vi "MSTAutoDailyReport.vi"() -> ()   [LabVIEW 2012]
uses:
  <vilib>/Utility/NIReport.llb/NI_report.lvclass
  <vilib>/addons/database/Connection.llb/DB Tools Open Connec (Path).vi
  <vilib>/addons/database/Connection.llb/Conn Execute.vi
  <vilib>/addons/database/Recordset.llb/Rec Fetch Recordset Data (R).vi
  <vilib>/addons/database/Recordset.llb/Rec Destroy - Connection.vi
  <vilib>/Utility/NIReport.llb/Append Text Table to Report (wrap).vi
  <vilib>/addons/database/_DB Variant To Data/Database Variant To Data.xnode
  <vilib>/addons/database/NI_Database_API.lvlib
  <vilib>/Utility/NIReport.llb/Excel/NI_Excel.lvclass
  <vilib>/addons/_office/NI_ReportGenerationToolkit.lvlib
panel:
  out "error out 3":errorcluster
  out "appended array 3":string[](array[string])
  out "recordset data 3":variant[][](array[variant])
  out "error out 5":errorcluster
  out "appended array 4":string[](array[string])
  out "recordset data 4":variant[][](array[variant])
  out "error out 6":errorcluster
  out "appended array 5":string[](array[string])
  out "recordset data 5":variant[][](array[variant])
  out "error out 4":errorcluster
  in  "Table Control 4":string[][](table)
  in  "Table Control 3":string[][](table)
  in  "Table Control 2":string[][](table)
  out "appended array":string[](array[string])
  out "recordset data":variant[][](array[variant])
  in  "Report Template":path=path "O:/Monitor/Report/MSTDailyReport.xls"
  in  "Table Control":string[][](table)
  out "error out":errorcluster
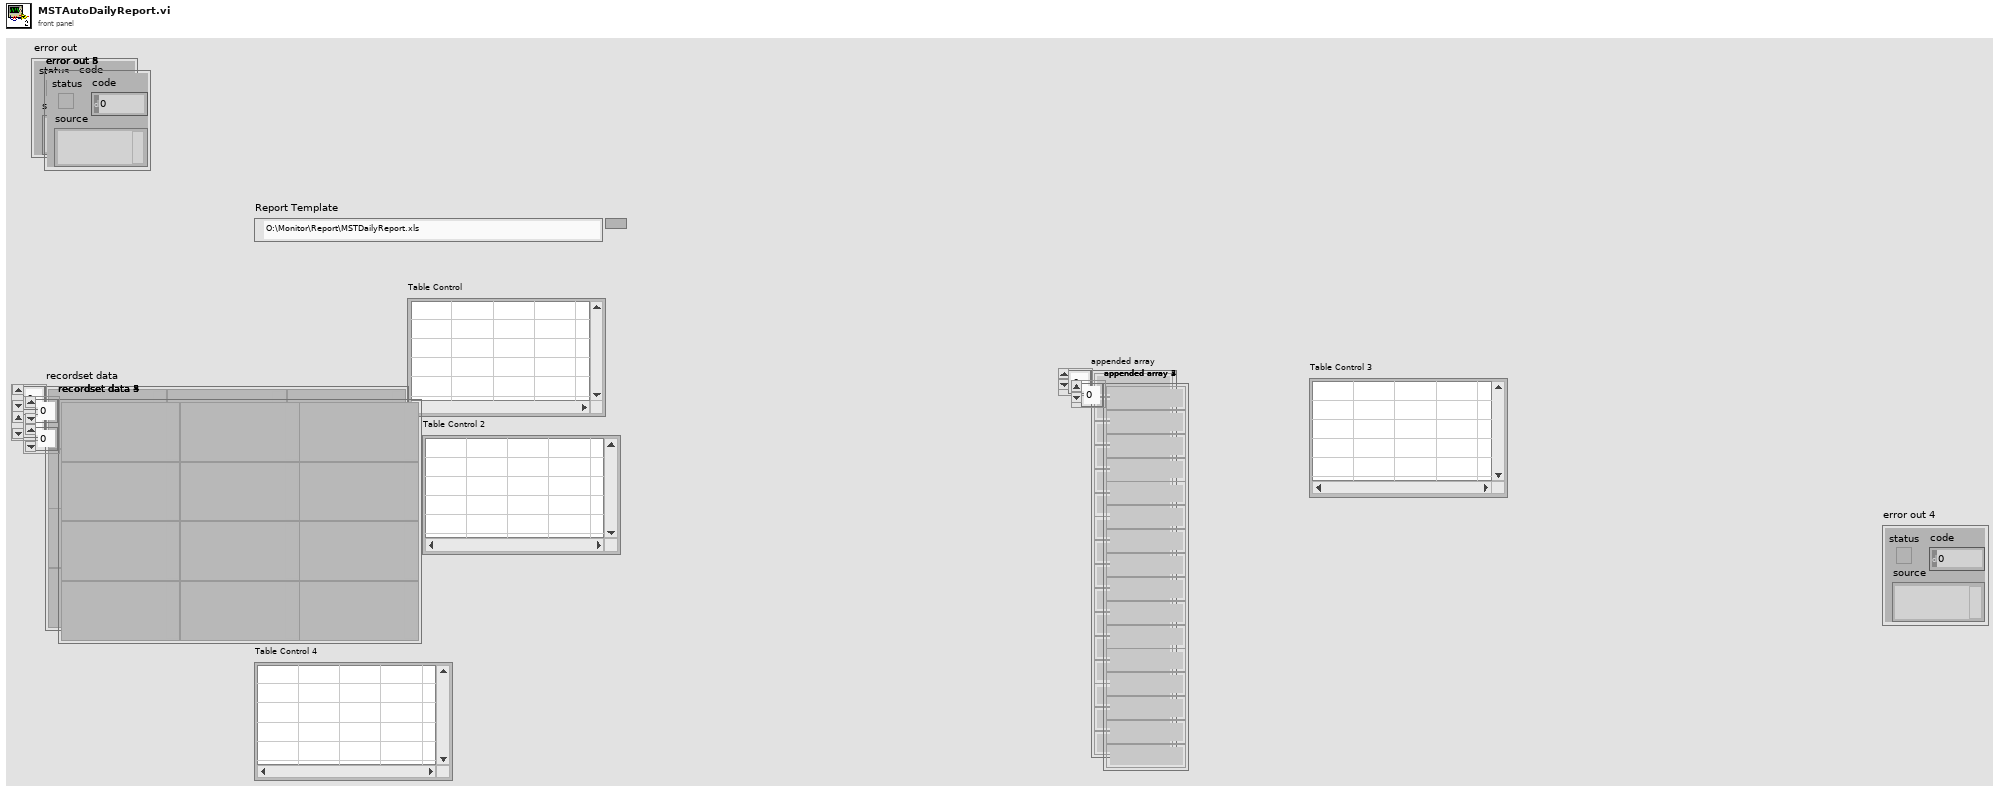
[diagram p1: front panel]
types:
  T1 = typedef "NI_Database_API.lvlib/Conn ObjectReference.ctl" = refnum<k1>
  T2 = typedef "NI_Database_API.lvlib/Rec ObjectReference.ctl" = refnum<k1>
  T3 = enum16{"Standard Report", "HTML", "Word", "Excel"}
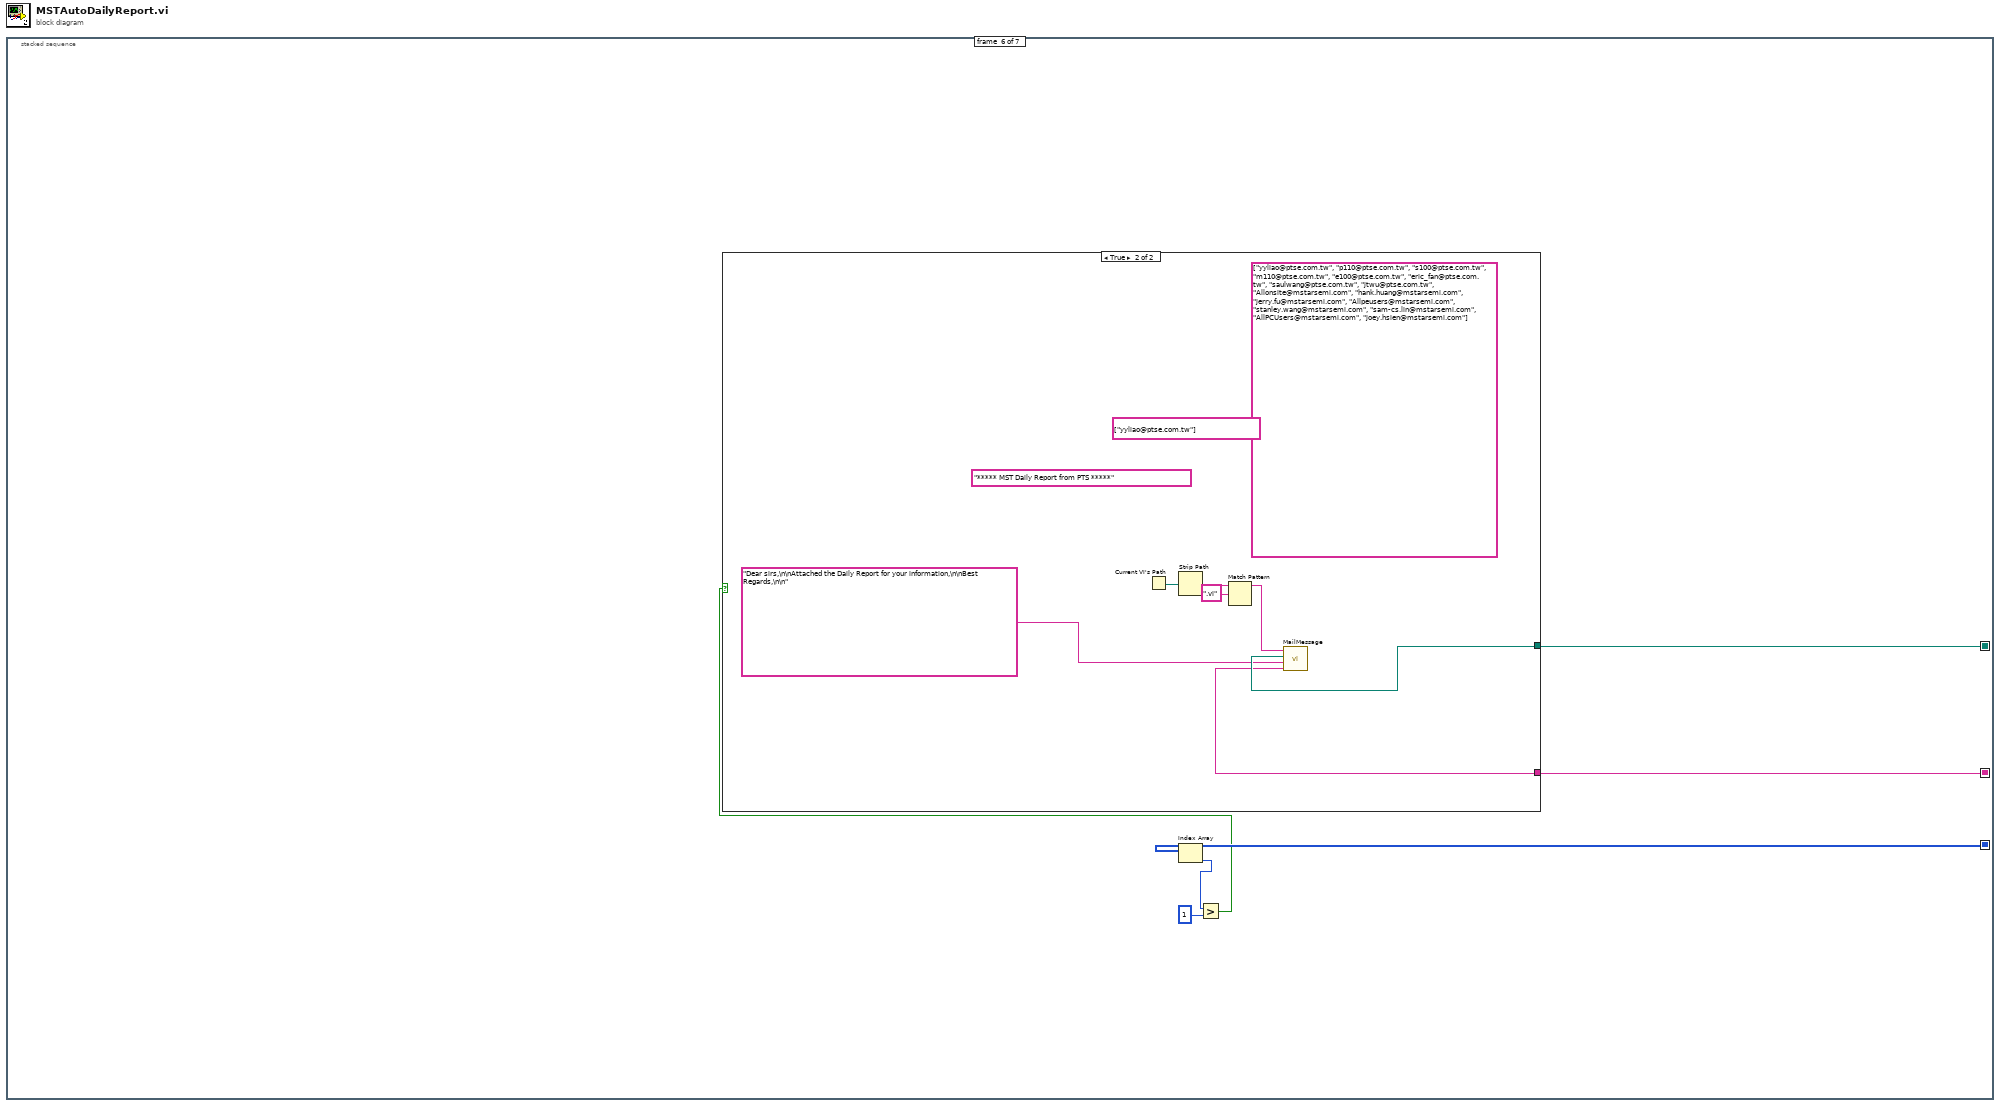
[diagram p0: block diagram]
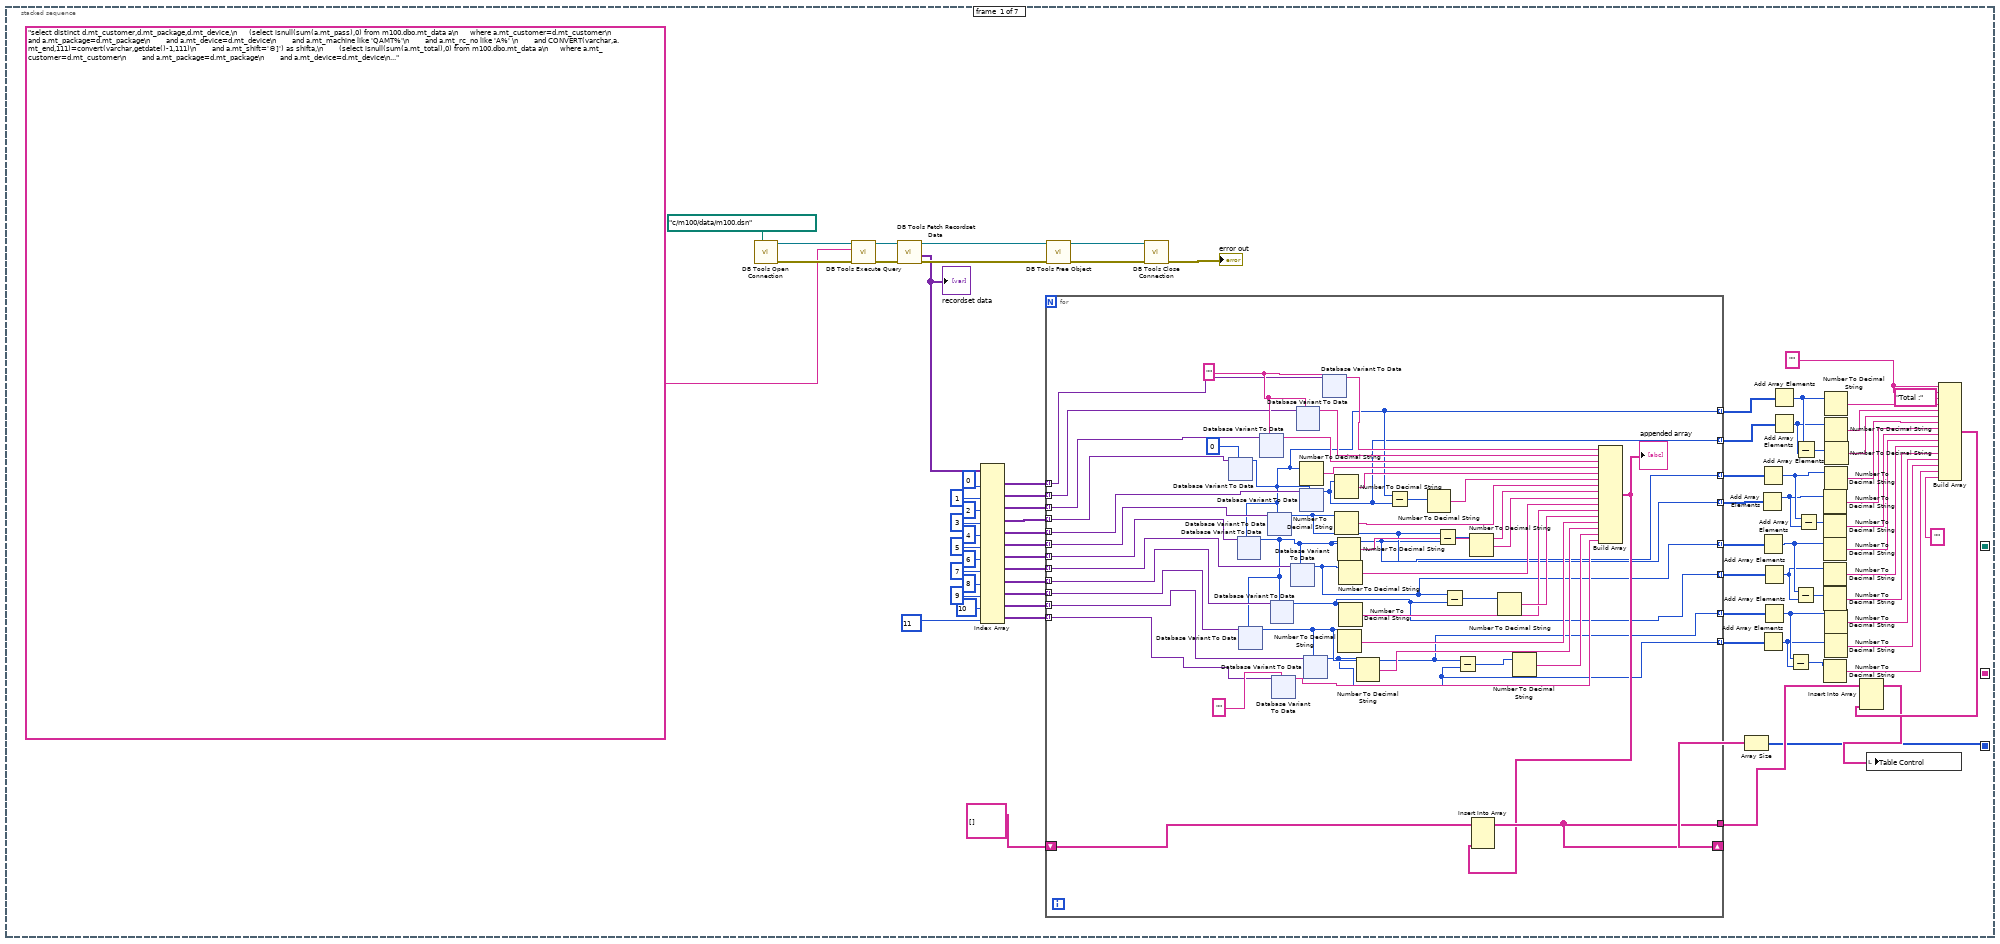
[diagram p2: hidden frame]
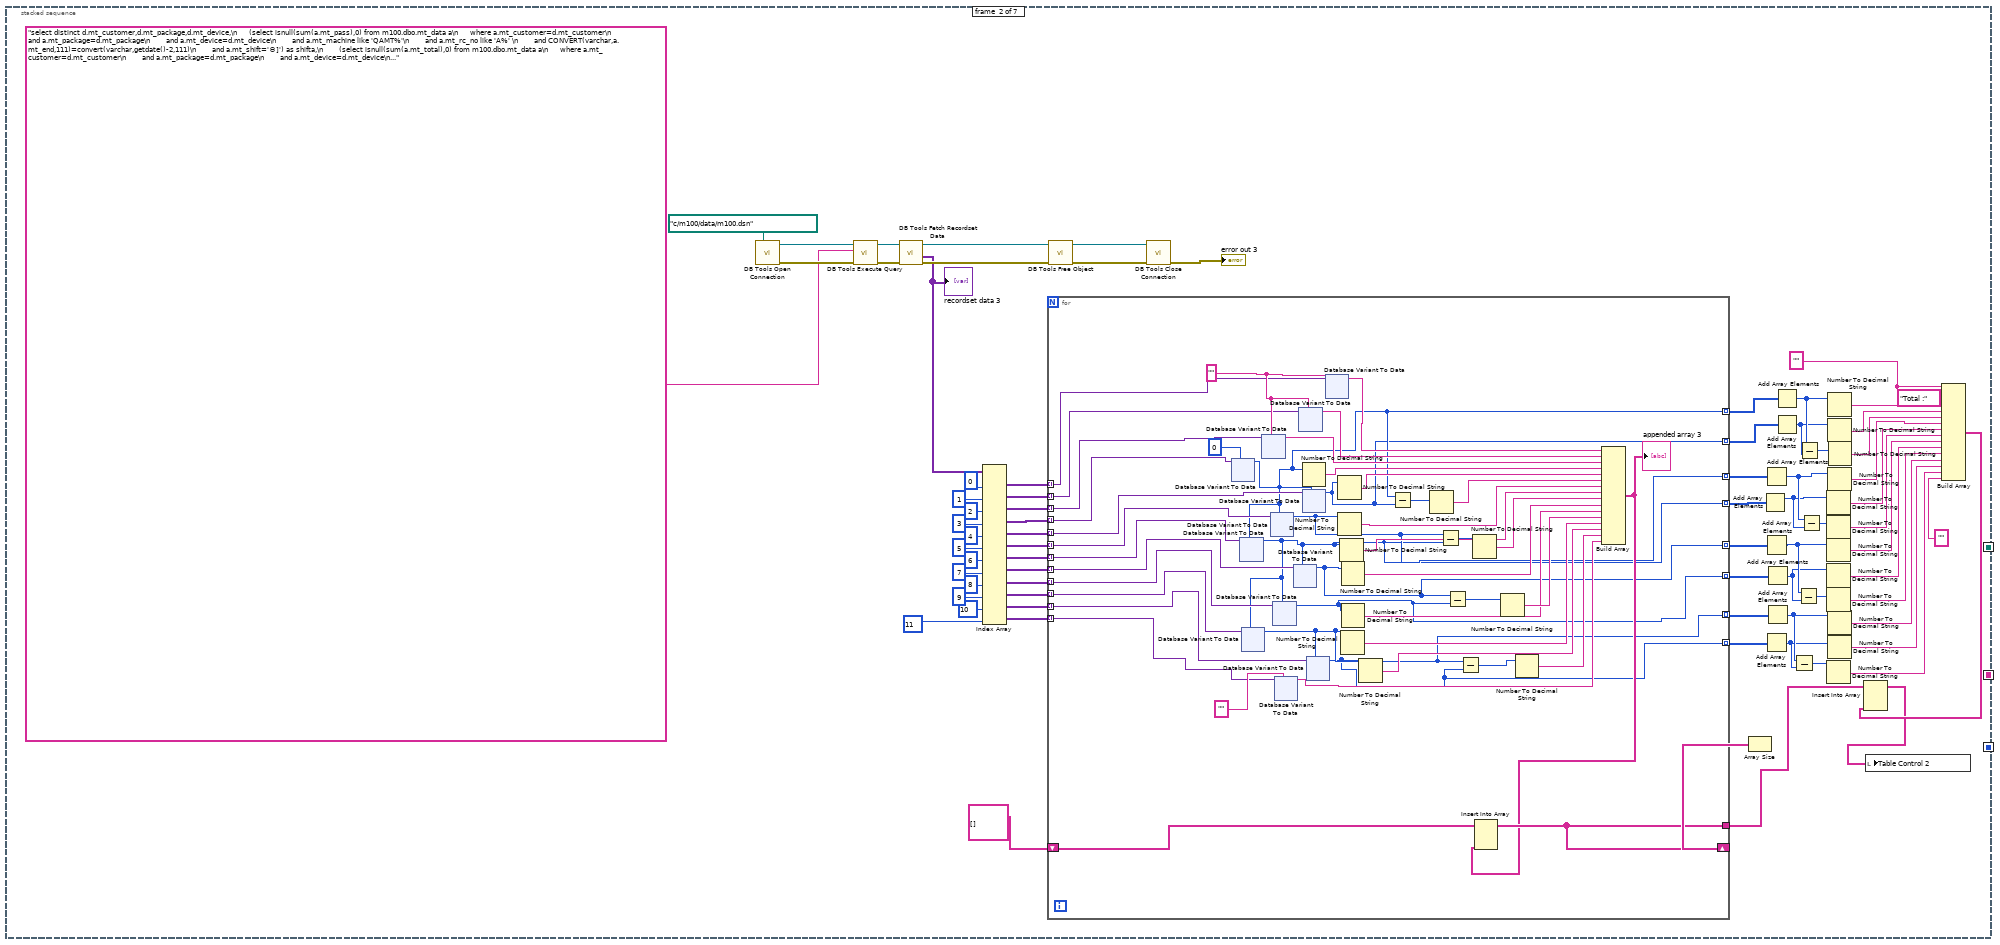
[diagram p3: hidden frame]
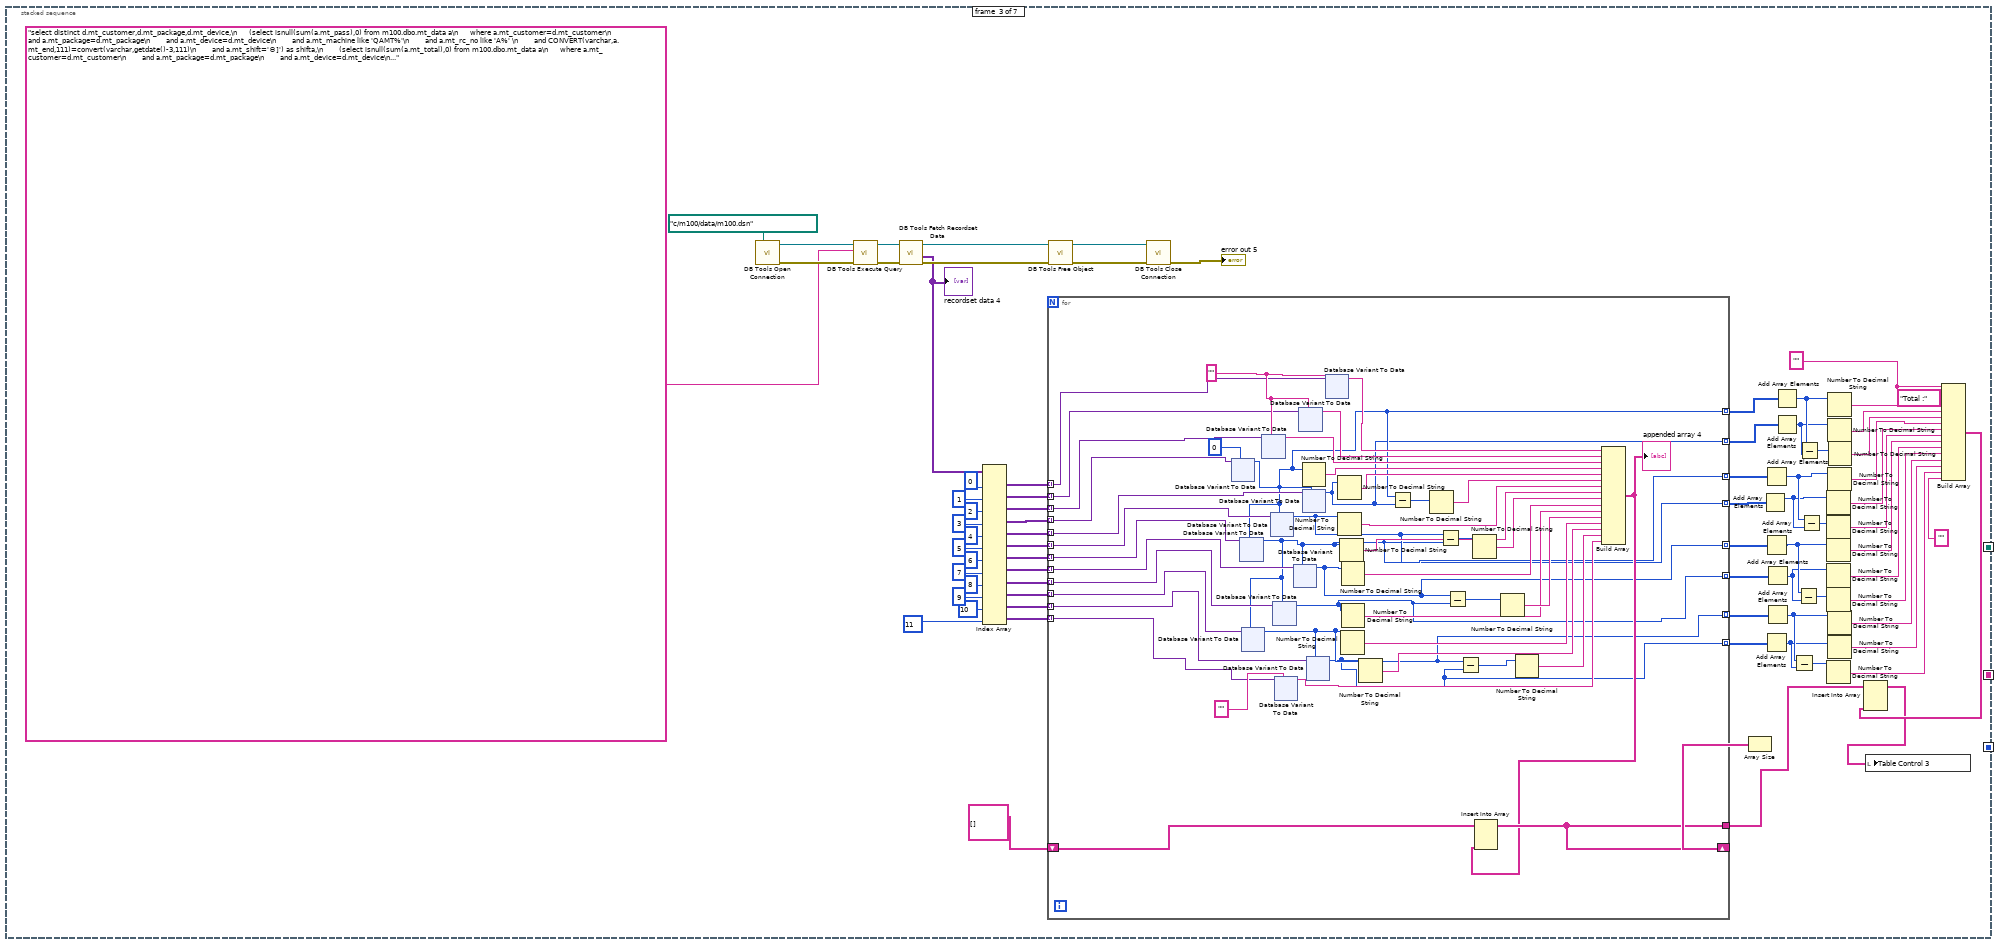
[diagram p4: hidden frame]
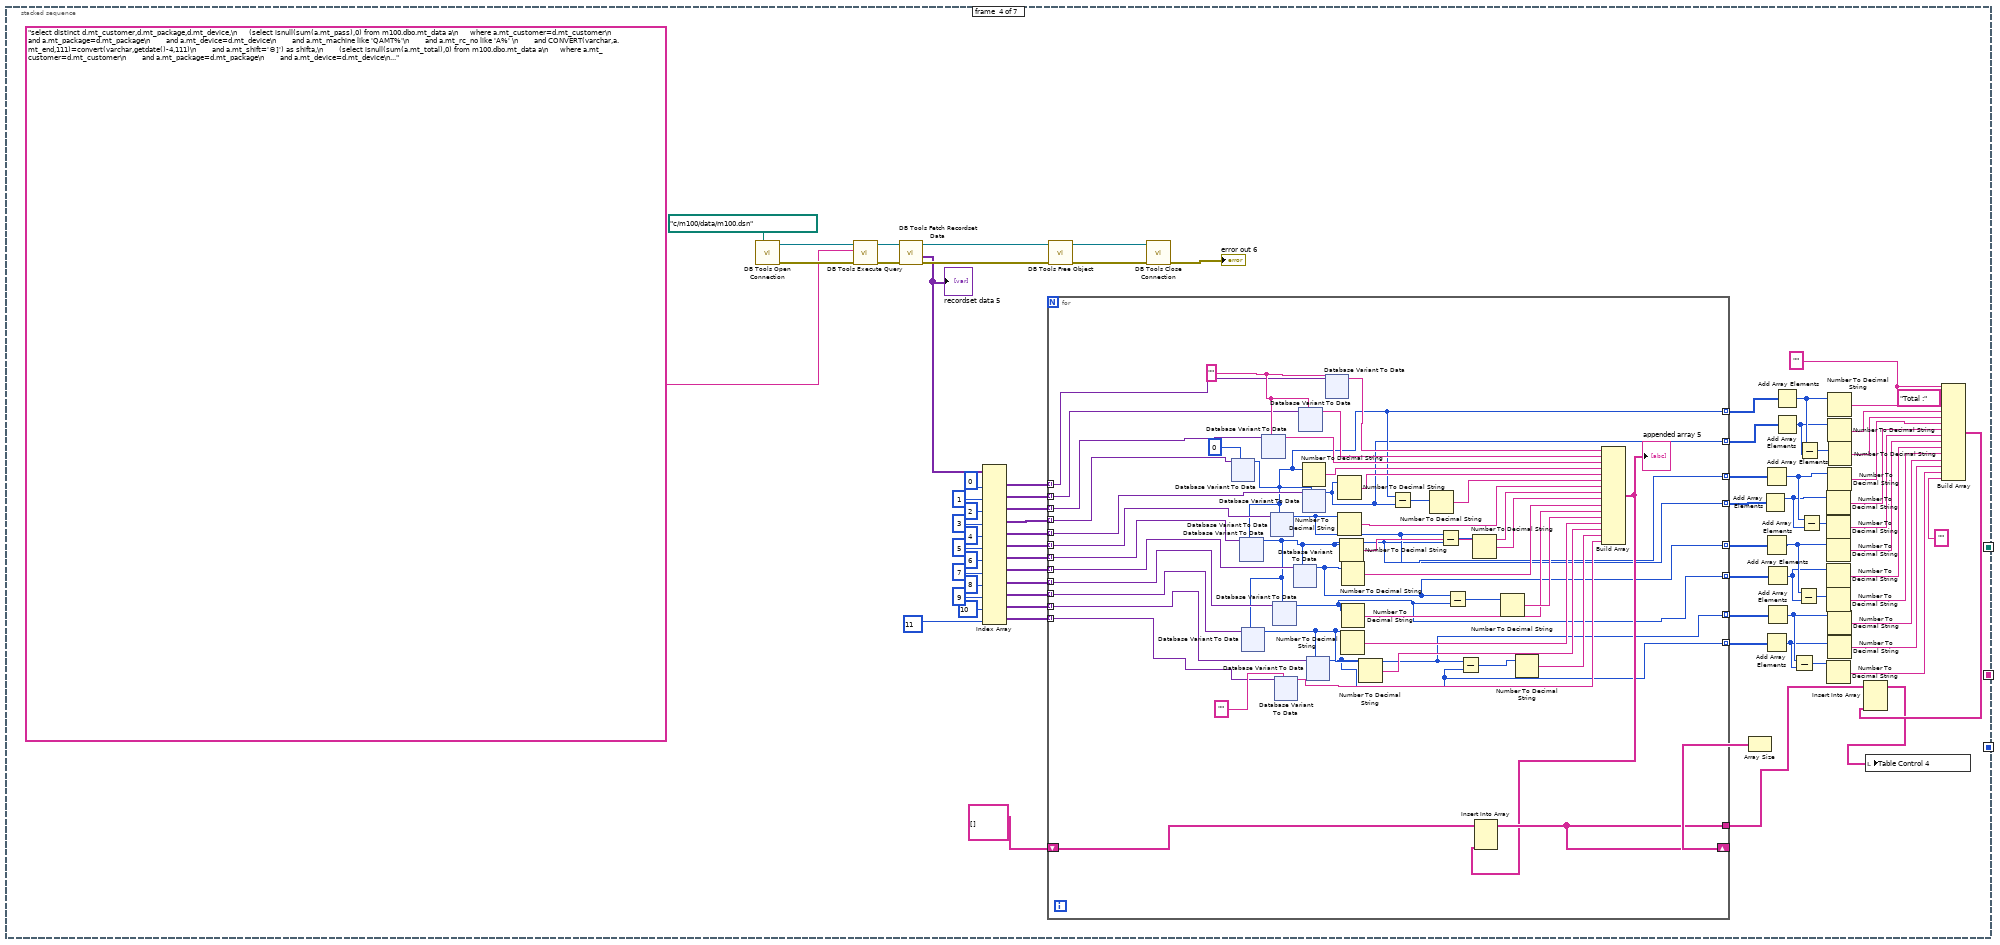
[diagram p5: hidden frame]
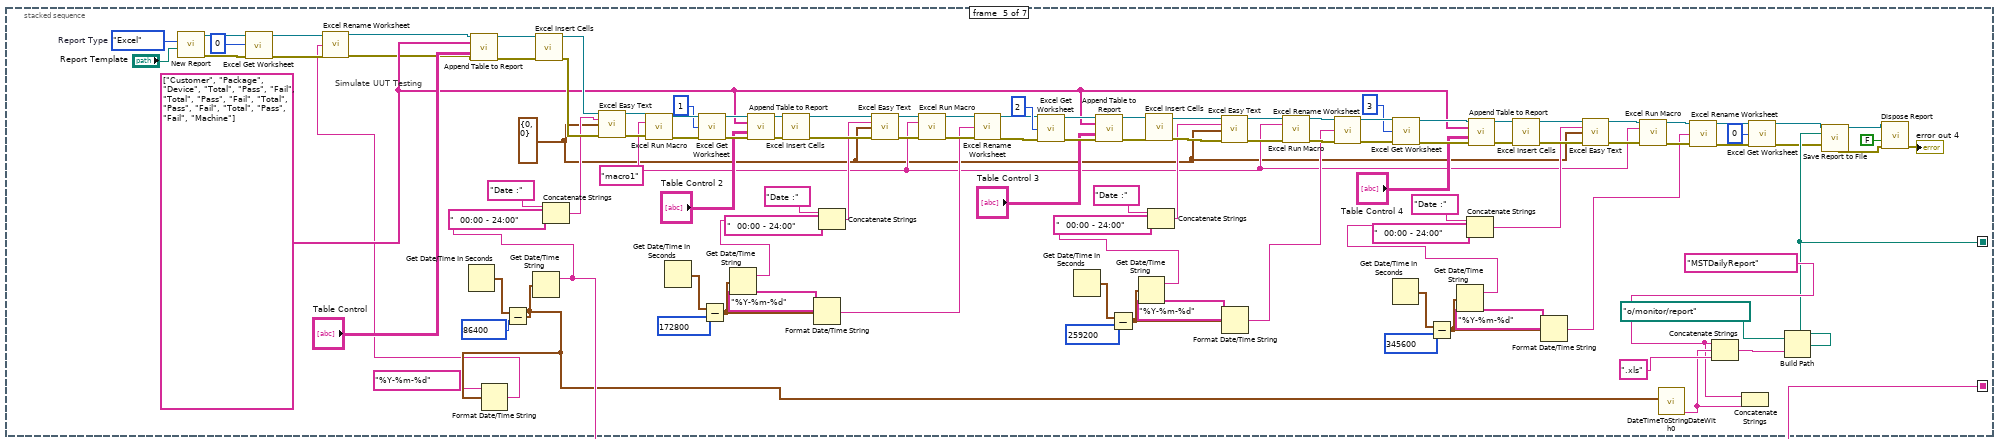
[diagram p6: hidden frame]
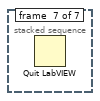
[diagram p8: hidden frame]
diagram:
  n1 = stacked-sequence {
    seq-local: [_ _ _ _ w2119 _ _] -> [_ _ _ _ _ w2143 _]
    seq-local: [_ _ _ _ w2118 _ _] -> [_ _ _ _ _ w2142 _]
    seq-local: [w1 _ _ _ _ _ _] -> [_ _ _ _ _ w2141 _]
    frame #0 {
      w37 = ""
      n2 = call-poly <vilib>:"DB Tools Open Connection.vi"("connection information"=path "c:/m100/data/m100.dsn") -> ("error out"=w72:errorcluster, "connection reference"=w76:T1)  [unwired: 7 in]
      n3 = call-poly <vilib>:"DB Tools Execute Query.vi"("error in (no error)"=w72, "SQL query"="select distinct d.mt_customer,d.mt_package,d.mt_device,\n      (select isnull(sum(a.mt_pass),0) from m100.dbo.mt_data a\n      where a.mt_customer=d.mt_customer\n        and a.mt_package=d.mt_package\n        and a.mt_device=d.mt_device\n        and a.mt_machine like 'QAMT%'\n        and a.mt_rc_no like 'A%' \n        and CONVERT(varchar,a.mt_end,111)=convert(varchar,getdate()-1,111)\n        and a.mt_shift='©]') as shifta,\n        (select isnull(sum(a.mt_total),0) from m100.dbo.mt_data a\n      where a.mt_customer=d.mt_customer\n        and a.mt_package=d.mt_package\n        and a.mt_device=d.mt_device\n        and a.mt_machine like 'QAMT%'\n        and a.mt_rc_no like 'A%' \n        and CONVERT(varchar,a.mt_end,111)=convert(varchar,getdate()-1,111)\n        and a.mt_shift='©]') as shifta1,\n        (select isnull(sum(b.mt_pass),0) from m100.dbo.mt_data b\n      where b.mt_customer=d.mt_customer\n        and b.mt_package=d.mt_package\n       and b.mt_device=d.mt_device\n        and b.mt_machine like 'QAMT%'\n        and b.mt_rc_no like 'A%' \n        and CONVERT(varchar,b.mt_end,111)=convert(varchar,getdate()-1,111)\n        and b.mt_shift='¦­') as shiftb,\n        (select isnull(sum(b.mt_total),0) from m100.dbo.mt_data b\n      where b.mt_customer=d.mt_customer\n        and b.mt_package=d.mt_package\n        and b.mt_device=d.mt_device\n        and b.mt_machine like 'QAMT%'\n        and b.mt_rc_no like 'A%' \n        and CONVERT(varchar,b.mt_end,111)=convert(varchar,getdate()-1,111)\n        and b.mt_shift='¦­') as shiftb1,\n        (select isnull(sum(c.mt_pass),0) from m100.dbo.mt_data c\n      where c.mt_customer=d.mt_customer\n        and c.mt_package=d.mt_package\n        and c.mt_device=d.mt_device\n        and c.mt_machine like 'QAMT%'\n        and c.mt_rc_no like 'A%' \n        and CONVERT(varchar,c.mt_end,111)=convert(varchar,getdate()-1,111)\n        and c.mt_shift='¤¤') as shiftc,\n        (select isnull(sum(c.mt_total),0) from m100.dbo.mt_data c\n      where c.mt_customer=d.mt_customer\n        and c.mt_package=d.mt_package\n        and c.mt_device=d.mt_device\n        and c.mt_machine like 'QAMT%'\n        and c.mt_rc_no like 'A%' \n        and CONVERT(varchar,c.mt_end,111)=convert(varchar,getdate()-1,111)\n        and c.mt_shift='¤¤') as shiftc1,\n        SUM(mt_pass),SUM(mt_total),master.dbo.GetEntityNameFromDateToDate(d.mt_customer,d.mt_package,d.mt_device,CONVERT(varchar,GETDATE()-1,111),CONVERT(varchar,GETDATE()-1,111))\n  FROM [m100].[dbo].[mt_data] d\n  WHERE d.mt_customer='MST'\n    and d.mt_machine like 'QAMT%'\n    AND CONVERT(varchar,d.mt_end,111)=convert(varchar,getdate()-1,111)\n    and d.mt_pass > 0 and d.mt_rc_no like 'A%'\n      group by d.mt_customer,d.mt_package,d.mt_device", "connection reference"=w76) -> ("error out"=w71:errorcluster, "recordset reference"=w75:T2)  [unwired: 5 in]
      n4 = call-poly <vilib>:"DB Tools Fetch Recordset Data.vi"("error in (no error)"=w71, "recordset reference"=w75) -> ("error out"=w70:errorcluster, "recordset data"=w40:variant[][], "recordset reference out"=w74:T2)  [unwired: 3 in]
      "recordset data" <- w40
      n5 = Index Array(array=w40, index (col) #1=0 ("index (row)"), index (col) #2=1 ("index (col)"), index (col) #3=2 ("disabled index (col)"), index (col) #4=3 ("index (col)"), index (col) #5=4 ("index (col)"), index (col) #6=5 ("index (col)"), index (col) #7=6 ("index (col)"), index (col) #8=7 ("index (col)"), index (col) #9=8 ("index (col)"), index (col) #10=9 ("index (col)"), index (col) #11=10 ("index (col)"), index (col) #12=11 ("index (col)")) -> (element #1=w44:variant[], element #2=w43:variant[], element #3=w57:variant[], element #4=w56:variant[], element #5=w55:variant[], element #6=w54:variant[], element #7=w53:variant[], element #8=w52:variant[], element #9=w51:variant[], element #10=w50:variant[], element #11=w49:variant[], element #12=w48:variant[])  [unwired: 12 in]
      n6 = for {
        tunnel: w57 -> [w96] mode=indexing
        tunnel: w56 -> [w95] mode=indexing
        tunnel: w55 -> [w94] mode=indexing
        tunnel: w54 -> [w93] mode=indexing
        tunnel: w53 -> [w92] mode=indexing
        tunnel: w52 -> [w91] mode=indexing
        tunnel: w51 -> [w90] mode=indexing
        tunnel: w50 -> [w89] mode=indexing
        tunnel: w49 -> [w88] mode=indexing
        tunnel: w48 -> [w87] mode=indexing
        tunnel: [w123] -> w30
        shift-right: [w123] -> w46
        shift-left: string[][] [] ("array") -> [w122]
        tunnel: w44 -> [w98] mode=indexing
        tunnel: w43 -> [w97] mode=indexing
        tunnel: [w85] -> w39 mode=indexing
        tunnel: [w84] -> w38 mode=indexing
        tunnel: [w83] -> w28 mode=indexing
        tunnel: [w82] -> w27 mode=indexing
        tunnel: [w81] -> w18 mode=indexing
        tunnel: [w80] -> w17 mode=indexing
        tunnel: [w79] -> w10 mode=indexing
        tunnel: [w78] -> w9 mode=indexing
        w121 = ""
        n7 = xnode "Database Variant To Data"("database variant"=w95, "type"=0) -> ("data"=w85:i32)  [unwired: 1 in, 1 out]
        n8 = xnode "Database Variant To Data"("database variant"=w92, "type"=w85) -> ("data"=w82:i32)  [unwired: 1 in, 1 out]
        n9 = xnode "Database Variant To Data"("database variant"=w89, "type"=w82) -> ("data"=w79:i32)  [unwired: 1 in, 1 out]
        n10 = xnode "Database Variant To Data"("database variant"=w96, "type"=w121) -> ("data"=w104:string)  [unwired: 1 in, 1 out]
        n11 = xnode "Database Variant To Data"("database variant"=w93, "type"=w85) -> ("data"=w83:i32)  [unwired: 1 in, 1 out]
        n12 = xnode "Database Variant To Data"("database variant"=w90, "type"=w82) -> ("data"=w80:i32)  [unwired: 1 in, 1 out]
        n13 = xnode "Database Variant To Data"("database variant"=w87, "type"="") -> ("data"=w116:string)  [unwired: 1 in, 1 out]
        n14 = xnode "Database Variant To Data"("database variant"=w91, "type"=w82) -> ("data"=w81:i32)  [unwired: 1 in, 1 out]
        n15 = xnode "Database Variant To Data"("database variant"=w97, "type"=w121) -> ("data"=w101:string)  [unwired: 1 in, 1 out]
        n16 = Number To Decimal String(number=w85) -> (decimal integer string=w103:string)  [unwired: 1 in]
        n17 = xnode "Database Variant To Data"("database variant"=w94, "type"=w85) -> ("data"=w84:i32)  [unwired: 1 in, 1 out]
        n18 = xnode "Database Variant To Data"("database variant"=w88, "type"=w79) -> ("data"=w78:i32)  [unwired: 1 in, 1 out]
        n19 = xnode "Database Variant To Data"("database variant"=w98, "type"=w121) -> ("data"=w105:string)  [unwired: 1 in, 1 out]
        n20 = Number To Decimal String(number=w84) -> (decimal integer string=w102:string)  [unwired: 1 in]
        n21 = Number To Decimal String(number=w83) -> (decimal integer string=w119:string)  [unwired: 1 in]
        n22 = Number To Decimal String(number=w82) -> (decimal integer string=w118:string)  [unwired: 1 in]
        n23 = Number To Decimal String(number=w79) -> (decimal integer string=w112:string)  [unwired: 1 in]
        n24 = Number To Decimal String(number=w81) -> (decimal integer string=w108:string)  [unwired: 1 in]
        n25 = Number To Decimal String(number=w80) -> (decimal integer string=w109:string)  [unwired: 1 in]
        n26 = Number To Decimal String(number=w78) -> (decimal integer string=w113:string)  [unwired: 1 in]
        n27 = Subtract(x=w85, y=w84) -> (x-y=w100:i32)
        n28 = Number To Decimal String(number=w100) -> (decimal integer string=w99:string)  [unwired: 1 in]
        n29 = Subtract(x=w83, y=w82) -> (x-y=w107:i32)
        n30 = Subtract(x=w81, y=w80) -> (x-y=w111:i32)
        n31 = Subtract(x=w79, y=w78) -> (x-y=w115:i32)
        n32 = Number To Decimal String(number=w107) -> (decimal integer string=w106:string)  [unwired: 1 in]
        n33 = Number To Decimal String(number=w111) -> (decimal integer string=w110:string)  [unwired: 1 in]
        n34 = Number To Decimal String(number=w115) -> (decimal integer string=w114:string)  [unwired: 1 in]
        n35 = Build Array(w105, w101, w104, w103, w102, w99, w119, w118, w106, w108, w109, w110, w112, w113, w114, w116) -> (w86:string[])
        "appended array" <- w86
        n36 = Insert Into Array(array=w122, new element=w86) -> (w123:string[][])  [unwired: 2 in]
      }
      n37 = call-poly <vilib>:"DB Tools Free Object.vi"("error in (no error)"=w70, "recordset reference"=w74) -> ("error out"=w69:errorcluster, "connection reference"=w73:T1)  [unwired: 8 in]
      n38 = call <vilib>:"DB Tools Close Connection.vi"("error in (no error)"=w69, "connection reference"=w73) -> ("error out"=→"error out":errorcluster)  [unwired: 5 in]
      n39 = Array Size(array=w46) -> (size(s)=w1:i32[])
      n40 = Add Array Elements(numeric array=w27) -> (sum=w21:i32)
      n41 = Add Array Elements(numeric array=w28) -> (sum=w22:i32)
      n42 = Add Array Elements(numeric array=w18) -> (sum=w14:i32)
      n43 = Add Array Elements(numeric array=w9) -> (sum=w7:i32)
      n44 = Add Array Elements(numeric array=w17) -> (sum=w13:i32)
      n45 = Add Array Elements(numeric array=w10) -> (sum=w8:i32)
      n46 = Add Array Elements(numeric array=w39) -> (sum=w34:i32)
      n47 = Add Array Elements(numeric array=w38) -> (sum=w33:i32)
      n48 = Subtract(x=w8, y=w7) -> (x-y=w6:i32)
      n49 = Subtract(x=w14, y=w13) -> (x-y=w11:i32)
      n50 = Subtract(x=w34, y=w33) -> (x-y=w26:i32)
      n51 = Subtract(x=w22, y=w21) -> (x-y=w19:i32)
      n52 = Number To Decimal String(number=w21) -> (decimal integer string=w23:string)  [unwired: 1 in]
      n53 = Number To Decimal String(number=w19) -> (decimal integer string=w20:string)  [unwired: 1 in]
      n54 = Number To Decimal String(number=w14) -> (decimal integer string=w16:string)  [unwired: 1 in]
      n55 = Number To Decimal String(number=w13) -> (decimal integer string=w15:string)  [unwired: 1 in]
      n56 = Number To Decimal String(number=w11) -> (decimal integer string=w12:string)  [unwired: 1 in]
      n57 = Number To Decimal String(number=w6) -> (decimal integer string=w3:string)  [unwired: 1 in]
      n58 = Number To Decimal String(number=w34) -> (decimal integer string=w36:string)  [unwired: 1 in]
      n59 = Number To Decimal String(number=w33) -> (decimal integer string=w35:string)  [unwired: 1 in]
      n60 = Number To Decimal String(number=w22) -> (decimal integer string=w25:string)  [unwired: 1 in]
      n61 = Number To Decimal String(number=w8) -> (decimal integer string=w5:string)  [unwired: 1 in]
      n62 = Number To Decimal String(number=w7) -> (decimal integer string=w4:string)  [unwired: 1 in]
      n63 = Number To Decimal String(number=w26) -> (decimal integer string=w32:string)  [unwired: 1 in]
      n64 = Build Array(w37, w37, "Total :" ("element"), w36, w35, w32, w25, w23, w20, w16, w15, w12, w5, w4, w3, "") -> (w31:string[])
      n65 = Insert Into Array(array=w30, new element=w31) -> (w29:string[][])  [unwired: 2 in]
      n66 = local write "Table Control"(w29) -> ()
    }
    frame #1 {
      w543 = ""
      n67 = call-poly <vilib>:"DB Tools Open Connection.vi"("connection information"=path "c:/m100/data/m100.dsn") -> ("error out"=w578:errorcluster, "connection reference"=w582:T1)  [unwired: 7 in]
      n68 = call-poly <vilib>:"DB Tools Execute Query.vi"("error in (no error)"=w578, "SQL query"="select distinct d.mt_customer,d.mt_package,d.mt_device,\n      (select isnull(sum(a.mt_pass),0) from m100.dbo.mt_data a\n      where a.mt_customer=d.mt_customer\n        and a.mt_package=d.mt_package\n        and a.mt_device=d.mt_device\n        and a.mt_machine like 'QAMT%'\n        and a.mt_rc_no like 'A%' \n        and CONVERT(varchar,a.mt_end,111)=convert(varchar,getdate()-2,111)\n        and a.mt_shift='©]') as shifta,\n        (select isnull(sum(a.mt_total),0) from m100.dbo.mt_data a\n      where a.mt_customer=d.mt_customer\n        and a.mt_package=d.mt_package\n        and a.mt_device=d.mt_device\n        and a.mt_machine like 'QAMT%'\n        and a.mt_rc_no like 'A%' \n        and CONVERT(varchar,a.mt_end,111)=convert(varchar,getdate()-2,111)\n        and a.mt_shift='©]') as shifta1,\n        (select isnull(sum(b.mt_pass),0) from m100.dbo.mt_data b\n      where b.mt_customer=d.mt_customer\n        and b.mt_package=d.mt_package\n       and b.mt_device=d.mt_device\n        and b.mt_machine like 'QAMT%'\n        and b.mt_rc_no like 'A%' \n        and CONVERT(varchar,b.mt_end,111)=convert(varchar,getdate()-2,111)\n        and b.mt_shift='¦­') as shiftb,\n        (select isnull(sum(b.mt_total),0) from m100.dbo.mt_data b\n      where b.mt_customer=d.mt_customer\n        and b.mt_package=d.mt_package\n        and b.mt_device=d.mt_device\n        and b.mt_machine like 'QAMT%'\n        and b.mt_rc_no like 'A%' \n        and CONVERT(varchar,b.mt_end,111)=convert(varchar,getdate()-2,111)\n        and b.mt_shift='¦­') as shiftb1,\n        (select isnull(sum(c.mt_pass),0) from m100.dbo.mt_data c\n      where c.mt_customer=d.mt_customer\n        and c.mt_package=d.mt_package\n        and c.mt_device=d.mt_device\n        and c.mt_machine like 'QAMT%'\n        and c.mt_rc_no like 'A%' \n        and CONVERT(varchar,c.mt_end,111)=convert(varchar,getdate()-2,111)\n        and c.mt_shift='¤¤') as shiftc,\n        (select isnull(sum(c.mt_total),0) from m100.dbo.mt_data c\n      where c.mt_customer=d.mt_customer\n        and c.mt_package=d.mt_package\n        and c.mt_device=d.mt_device\n        and c.mt_machine like 'QAMT%'\n        and c.mt_rc_no like 'A%' \n        and CONVERT(varchar,c.mt_end,111)=convert(varchar,getdate()-2,111)\n        and c.mt_shift='¤¤') as shiftc1,\n        SUM(mt_pass),SUM(mt_total),master.dbo.GetEntityNameFromDateToDate(d.mt_customer,d.mt_package,d.mt_device,CONVERT(varchar,GETDATE()-2,111),CONVERT(varchar,GETDATE()-2,111))\n  FROM [m100].[dbo].[mt_data] d\n  WHERE d.mt_customer='MST'\n    and d.mt_machine like 'QAMT%'\n    AND CONVERT(varchar,d.mt_end,111)=convert(varchar,getdate()-2,111)\n    and d.mt_pass > 0 and d.mt_rc_no like 'A%'\n      group by d.mt_customer,d.mt_package,d.mt_device", "connection reference"=w582) -> ("error out"=w577:errorcluster, "recordset reference"=w581:T2)  [unwired: 5 in]
      n69 = call-poly <vilib>:"DB Tools Fetch Recordset Data.vi"("error in (no error)"=w577, "recordset reference"=w581) -> ("error out"=w576:errorcluster, "recordset data"=w546:variant[][], "recordset reference out"=w580:T2)  [unwired: 3 in]
      "recordset data 3" <- w546
      n70 = Index Array(array=w546, index (col) #1=0 ("index (row)"), index (col) #2=1 ("index (col)"), index (col) #3=2 ("disabled index (col)"), index (col) #4=3 ("index (col)"), index (col) #5=4 ("index (col)"), index (col) #6=5 ("index (col)"), index (col) #7=6 ("index (col)"), index (col) #8=7 ("index (col)"), index (col) #9=8 ("index (col)"), index (col) #10=9 ("index (col)"), index (col) #11=10 ("index (col)"), index (col) #12=11 ("index (col)")) -> (element #1=w550:variant[], element #2=w549:variant[], element #3=w563:variant[], element #4=w562:variant[], element #5=w561:variant[], element #6=w560:variant[], element #7=w559:variant[], element #8=w558:variant[], element #9=w557:variant[], element #10=w556:variant[], element #11=w555:variant[], element #12=w554:variant[])  [unwired: 12 in]
      n71 = for {
        tunnel: w563 -> [w602] mode=indexing
        tunnel: w562 -> [w601] mode=indexing
        tunnel: w561 -> [w600] mode=indexing
        tunnel: w560 -> [w599] mode=indexing
        tunnel: w559 -> [w598] mode=indexing
        tunnel: w558 -> [w597] mode=indexing
        tunnel: w557 -> [w596] mode=indexing
        tunnel: w556 -> [w595] mode=indexing
        tunnel: w555 -> [w594] mode=indexing
        tunnel: w554 -> [w593] mode=indexing
        tunnel: [w629] -> w536
        shift-right: [w629] -> w552
        shift-left: string[][] [] ("array") -> [w628]
        tunnel: w550 -> [w604] mode=indexing
        tunnel: w549 -> [w603] mode=indexing
        tunnel: [w591] -> w545 mode=indexing
        tunnel: [w590] -> w544 mode=indexing
        tunnel: [w589] -> w534 mode=indexing
        tunnel: [w588] -> w533 mode=indexing
        tunnel: [w587] -> w524 mode=indexing
        tunnel: [w586] -> w523 mode=indexing
        tunnel: [w585] -> w516 mode=indexing
        tunnel: [w584] -> w515 mode=indexing
        w627 = ""
        n72 = xnode "Database Variant To Data"("database variant"=w601, "type"=0) -> ("data"=w591:i32)  [unwired: 1 in, 1 out]
        n73 = xnode "Database Variant To Data"("database variant"=w598, "type"=w591) -> ("data"=w588:i32)  [unwired: 1 in, 1 out]
        n74 = xnode "Database Variant To Data"("database variant"=w595, "type"=w588) -> ("data"=w585:i32)  [unwired: 1 in, 1 out]
        n75 = xnode "Database Variant To Data"("database variant"=w602, "type"=w627) -> ("data"=w610:string)  [unwired: 1 in, 1 out]
        n76 = xnode "Database Variant To Data"("database variant"=w599, "type"=w591) -> ("data"=w589:i32)  [unwired: 1 in, 1 out]
        n77 = xnode "Database Variant To Data"("database variant"=w596, "type"=w588) -> ("data"=w586:i32)  [unwired: 1 in, 1 out]
        n78 = xnode "Database Variant To Data"("database variant"=w593, "type"="") -> ("data"=w622:string)  [unwired: 1 in, 1 out]
        n79 = xnode "Database Variant To Data"("database variant"=w597, "type"=w588) -> ("data"=w587:i32)  [unwired: 1 in, 1 out]
        n80 = xnode "Database Variant To Data"("database variant"=w603, "type"=w627) -> ("data"=w607:string)  [unwired: 1 in, 1 out]
        n81 = Number To Decimal String(number=w591) -> (decimal integer string=w609:string)  [unwired: 1 in]
        n82 = xnode "Database Variant To Data"("database variant"=w600, "type"=w591) -> ("data"=w590:i32)  [unwired: 1 in, 1 out]
        n83 = xnode "Database Variant To Data"("database variant"=w594, "type"=w585) -> ("data"=w584:i32)  [unwired: 1 in, 1 out]
        n84 = xnode "Database Variant To Data"("database variant"=w604, "type"=w627) -> ("data"=w611:string)  [unwired: 1 in, 1 out]
        n85 = Number To Decimal String(number=w590) -> (decimal integer string=w608:string)  [unwired: 1 in]
        n86 = Number To Decimal String(number=w589) -> (decimal integer string=w625:string)  [unwired: 1 in]
        n87 = Number To Decimal String(number=w588) -> (decimal integer string=w624:string)  [unwired: 1 in]
        n88 = Number To Decimal String(number=w585) -> (decimal integer string=w618:string)  [unwired: 1 in]
        n89 = Number To Decimal String(number=w587) -> (decimal integer string=w614:string)  [unwired: 1 in]
        n90 = Number To Decimal String(number=w586) -> (decimal integer string=w615:string)  [unwired: 1 in]
        n91 = Number To Decimal String(number=w584) -> (decimal integer string=w619:string)  [unwired: 1 in]
        n92 = Subtract(x=w591, y=w590) -> (x-y=w606:i32)
        n93 = Number To Decimal String(number=w606) -> (decimal integer string=w605:string)  [unwired: 1 in]
        n94 = Subtract(x=w589, y=w588) -> (x-y=w613:i32)
        n95 = Subtract(x=w587, y=w586) -> (x-y=w617:i32)
        n96 = Subtract(x=w585, y=w584) -> (x-y=w621:i32)
        n97 = Number To Decimal String(number=w613) -> (decimal integer string=w612:string)  [unwired: 1 in]
        n98 = Number To Decimal String(number=w617) -> (decimal integer string=w616:string)  [unwired: 1 in]
        n99 = Number To Decimal String(number=w621) -> (decimal integer string=w620:string)  [unwired: 1 in]
        n100 = Build Array(w611, w607, w610, w609, w608, w605, w625, w624, w612, w614, w615, w616, w618, w619, w620, w622) -> (w592:string[])
        "appended array 3" <- w592
        n101 = Insert Into Array(array=w628, new element=w592) -> (w629:string[][])  [unwired: 2 in]
      }
      n102 = call-poly <vilib>:"DB Tools Free Object.vi"("error in (no error)"=w576, "recordset reference"=w580) -> ("error out"=w575:errorcluster, "connection reference"=w579:T1)  [unwired: 8 in]
      n103 = call <vilib>:"DB Tools Close Connection.vi"("error in (no error)"=w575, "connection reference"=w579) -> ("error out"=→"error out 3":errorcluster)  [unwired: 5 in]
      n104 = Array Size(array=w552) -> ()  [unwired: 1 out]
      n105 = Add Array Elements(numeric array=w533) -> (sum=w527:i32)
      n106 = Add Array Elements(numeric array=w534) -> (sum=w528:i32)
      n107 = Add Array Elements(numeric array=w524) -> (sum=w520:i32)
      n108 = Add Array Elements(numeric array=w515) -> (sum=w513:i32)
      n109 = Add Array Elements(numeric array=w523) -> (sum=w519:i32)
      n110 = Add Array Elements(numeric array=w516) -> (sum=w514:i32)
      n111 = Add Array Elements(numeric array=w545) -> (sum=w540:i32)
      n112 = Add Array Elements(numeric array=w544) -> (sum=w539:i32)
      n113 = Subtract(x=w514, y=w513) -> (x-y=w512:i32)
      n114 = Subtract(x=w520, y=w519) -> (x-y=w517:i32)
      n115 = Subtract(x=w540, y=w539) -> (x-y=w532:i32)
      n116 = Subtract(x=w528, y=w527) -> (x-y=w525:i32)
      n117 = Number To Decimal String(number=w527) -> (decimal integer string=w529:string)  [unwired: 1 in]
      n118 = Number To Decimal String(number=w525) -> (decimal integer string=w526:string)  [unwired: 1 in]
      n119 = Number To Decimal String(number=w520) -> (decimal integer string=w522:string)  [unwired: 1 in]
      n120 = Number To Decimal String(number=w519) -> (decimal integer string=w521:string)  [unwired: 1 in]
      n121 = Number To Decimal String(number=w517) -> (decimal integer string=w518:string)  [unwired: 1 in]
      n122 = Number To Decimal String(number=w512) -> (decimal integer string=w509:string)  [unwired: 1 in]
      n123 = Number To Decimal String(number=w540) -> (decimal integer string=w542:string)  [unwired: 1 in]
      n124 = Number To Decimal String(number=w539) -> (decimal integer string=w541:string)  [unwired: 1 in]
      n125 = Number To Decimal String(number=w528) -> (decimal integer string=w531:string)  [unwired: 1 in]
      n126 = Number To Decimal String(number=w514) -> (decimal integer string=w511:string)  [unwired: 1 in]
      n127 = Number To Decimal String(number=w513) -> (decimal integer string=w510:string)  [unwired: 1 in]
      n128 = Number To Decimal String(number=w532) -> (decimal integer string=w538:string)  [unwired: 1 in]
      n129 = Build Array(w543, w543, "Total :" ("element"), w542, w541, w538, w531, w529, w526, w522, w521, w518, w511, w510, w509, "") -> (w537:string[])
      n130 = Insert Into Array(array=w536, new element=w537) -> (w535:string[][])  [unwired: 2 in]
      n131 = local write "Table Control 2"(w535) -> ()
    }
    frame #2 {
      w1049 = ""
      n132 = call-poly <vilib>:"DB Tools Open Connection.vi"("connection information"=path "c:/m100/data/m100.dsn") -> ("error out"=w1084:errorcluster, "connection reference"=w1088:T1)  [unwired: 7 in]
      n133 = call-poly <vilib>:"DB Tools Execute Query.vi"("error in (no error)"=w1084, "SQL query"="select distinct d.mt_customer,d.mt_package,d.mt_device,\n      (select isnull(sum(a.mt_pass),0) from m100.dbo.mt_data a\n      where a.mt_customer=d.mt_customer\n        and a.mt_package=d.mt_package\n        and a.mt_device=d.mt_device\n        and a.mt_machine like 'QAMT%'\n        and a.mt_rc_no like 'A%' \n        and CONVERT(varchar,a.mt_end,111)=convert(varchar,getdate()-3,111)\n        and a.mt_shift='©]') as shifta,\n        (select isnull(sum(a.mt_total),0) from m100.dbo.mt_data a\n      where a.mt_customer=d.mt_customer\n        and a.mt_package=d.mt_package\n        and a.mt_device=d.mt_device\n        and a.mt_machine like 'QAMT%'\n        and a.mt_rc_no like 'A%' \n        and CONVERT(varchar,a.mt_end,111)=convert(varchar,getdate()-3,111)\n        and a.mt_shift='©]') as shifta1,\n        (select isnull(sum(b.mt_pass),0) from m100.dbo.mt_data b\n      where b.mt_customer=d.mt_customer\n        and b.mt_package=d.mt_package\n       and b.mt_device=d.mt_device\n        and b.mt_machine like 'QAMT%'\n        and b.mt_rc_no like 'A%' \n        and CONVERT(varchar,b.mt_end,111)=convert(varchar,getdate()-3,111)\n        and b.mt_shift='¦­') as shiftb,\n        (select isnull(sum(b.mt_total),0) from m100.dbo.mt_data b\n      where b.mt_customer=d.mt_customer\n        and b.mt_package=d.mt_package\n        and b.mt_device=d.mt_device\n        and b.mt_machine like 'QAMT%'\n        and b.mt_rc_no like 'A%' \n        and CONVERT(varchar,b.mt_end,111)=convert(varchar,getdate()-3,111)\n        and b.mt_shift='¦­') as shiftb1,\n        (select isnull(sum(c.mt_pass),0) from m100.dbo.mt_data c\n      where c.mt_customer=d.mt_customer\n        and c.mt_package=d.mt_package\n        and c.mt_device=d.mt_device\n        and c.mt_machine like 'QAMT%'\n        and c.mt_rc_no like 'A%' \n        and CONVERT(varchar,c.mt_end,111)=convert(varchar,getdate()-3,111)\n        and c.mt_shift='¤¤') as shiftc,\n        (select isnull(sum(c.mt_total),0) from m100.dbo.mt_data c\n      where c.mt_customer=d.mt_customer\n        and c.mt_package=d.mt_package\n        and c.mt_device=d.mt_device\n        and c.mt_machine like 'QAMT%'\n        and c.mt_rc_no like 'A%' \n        and CONVERT(varchar,c.mt_end,111)=convert(varchar,getdate()-3,111)\n        and c.mt_shift='¤¤') as shiftc1,\n        SUM(mt_pass),SUM(mt_total),master.dbo.GetEntityNameFromDateToDate(d.mt_customer,d.mt_package,d.mt_device,CONVERT(varchar,GETDATE()-3,111),CONVERT(varchar,GETDATE()-3,111))\n  FROM [m100].[dbo].[mt_data] d\n  WHERE d.mt_customer='MST'\n    and d.mt_machine like 'QAMT%'\n    AND CONVERT(varchar,d.mt_end,111)=convert(varchar,getdate()-3,111)\n    and d.mt_pass > 0 and d.mt_rc_no like 'A%'\n      group by d.mt_customer,d.mt_package,d.mt_device", "connection reference"=w1088) -> ("error out"=w1083:errorcluster, "recordset reference"=w1087:T2)  [unwired: 5 in]
      n134 = call-poly <vilib>:"DB Tools Fetch Recordset Data.vi"("error in (no error)"=w1083, "recordset reference"=w1087) -> ("error out"=w1082:errorcluster, "recordset data"=w1052:variant[][], "recordset reference out"=w1086:T2)  [unwired: 3 in]
      "recordset data 4" <- w1052
      n135 = Index Array(array=w1052, index (col) #1=0 ("index (row)"), index (col) #2=1 ("index (col)"), index (col) #3=2 ("disabled index (col)"), index (col) #4=3 ("index (col)"), index (col) #5=4 ("index (col)"), index (col) #6=5 ("index (col)"), index (col) #7=6 ("index (col)"), index (col) #8=7 ("index (col)"), index (col) #9=8 ("index (col)"), index (col) #10=9 ("index (col)"), index (col) #11=10 ("index (col)"), index (col) #12=11 ("index (col)")) -> (element #1=w1056:variant[], element #2=w1055:variant[], element #3=w1069:variant[], element #4=w1068:variant[], element #5=w1067:variant[], element #6=w1066:variant[], element #7=w1065:variant[], element #8=w1064:variant[], element #9=w1063:variant[], element #10=w1062:variant[], element #11=w1061:variant[], element #12=w1060:variant[])  [unwired: 12 in]
      n136 = for {
        tunnel: w1069 -> [w1108] mode=indexing
        tunnel: w1068 -> [w1107] mode=indexing
        tunnel: w1067 -> [w1106] mode=indexing
        tunnel: w1066 -> [w1105] mode=indexing
        tunnel: w1065 -> [w1104] mode=indexing
        tunnel: w1064 -> [w1103] mode=indexing
        tunnel: w1063 -> [w1102] mode=indexing
        tunnel: w1062 -> [w1101] mode=indexing
        tunnel: w1061 -> [w1100] mode=indexing
        tunnel: w1060 -> [w1099] mode=indexing
        tunnel: [w1135] -> w1042
        shift-right: [w1135] -> w1058
        shift-left: string[][] [] ("array") -> [w1134]
        tunnel: w1056 -> [w1110] mode=indexing
        tunnel: w1055 -> [w1109] mode=indexing
        tunnel: [w1097] -> w1051 mode=indexing
        tunnel: [w1096] -> w1050 mode=indexing
        tunnel: [w1095] -> w1040 mode=indexing
        tunnel: [w1094] -> w1039 mode=indexing
        tunnel: [w1093] -> w1030 mode=indexing
        tunnel: [w1092] -> w1029 mode=indexing
        tunnel: [w1091] -> w1022 mode=indexing
        tunnel: [w1090] -> w1021 mode=indexing
        w1133 = ""
        n137 = xnode "Database Variant To Data"("database variant"=w1107, "type"=0) -> ("data"=w1097:i32)  [unwired: 1 in, 1 out]
        n138 = xnode "Database Variant To Data"("database variant"=w1104, "type"=w1097) -> ("data"=w1094:i32)  [unwired: 1 in, 1 out]
        n139 = xnode "Database Variant To Data"("database variant"=w1101, "type"=w1094) -> ("data"=w1091:i32)  [unwired: 1 in, 1 out]
        n140 = xnode "Database Variant To Data"("database variant"=w1108, "type"=w1133) -> ("data"=w1116:string)  [unwired: 1 in, 1 out]
        n141 = xnode "Database Variant To Data"("database variant"=w1105, "type"=w1097) -> ("data"=w1095:i32)  [unwired: 1 in, 1 out]
        n142 = xnode "Database Variant To Data"("database variant"=w1102, "type"=w1094) -> ("data"=w1092:i32)  [unwired: 1 in, 1 out]
        n143 = xnode "Database Variant To Data"("database variant"=w1099, "type"="") -> ("data"=w1128:string)  [unwired: 1 in, 1 out]
        n144 = xnode "Database Variant To Data"("database variant"=w1103, "type"=w1094) -> ("data"=w1093:i32)  [unwired: 1 in, 1 out]
        n145 = xnode "Database Variant To Data"("database variant"=w1109, "type"=w1133) -> ("data"=w1113:string)  [unwired: 1 in, 1 out]
        n146 = Number To Decimal String(number=w1097) -> (decimal integer string=w1115:string)  [unwired: 1 in]
        n147 = xnode "Database Variant To Data"("database variant"=w1106, "type"=w1097) -> ("data"=w1096:i32)  [unwired: 1 in, 1 out]
        n148 = xnode "Database Variant To Data"("database variant"=w1100, "type"=w1091) -> ("data"=w1090:i32)  [unwired: 1 in, 1 out]
        n149 = xnode "Database Variant To Data"("database variant"=w1110, "type"=w1133) -> ("data"=w1117:string)  [unwired: 1 in, 1 out]
        n150 = Number To Decimal String(number=w1096) -> (decimal integer string=w1114:string)  [unwired: 1 in]
        n151 = Number To Decimal String(number=w1095) -> (decimal integer string=w1131:string)  [unwired: 1 in]
        n152 = Number To Decimal String(number=w1094) -> (decimal integer string=w1130:string)  [unwired: 1 in]
        n153 = Number To Decimal String(number=w1091) -> (decimal integer string=w1124:string)  [unwired: 1 in]
        n154 = Number To Decimal String(number=w1093) -> (decimal integer string=w1120:string)  [unwired: 1 in]
        n155 = Number To Decimal String(number=w1092) -> (decimal integer string=w1121:string)  [unwired: 1 in]
        n156 = Number To Decimal String(number=w1090) -> (decimal integer string=w1125:string)  [unwired: 1 in]
        n157 = Subtract(x=w1097, y=w1096) -> (x-y=w1112:i32)
        n158 = Number To Decimal String(number=w1112) -> (decimal integer string=w1111:string)  [unwired: 1 in]
        n159 = Subtract(x=w1095, y=w1094) -> (x-y=w1119:i32)
        n160 = Subtract(x=w1093, y=w1092) -> (x-y=w1123:i32)
        n161 = Subtract(x=w1091, y=w1090) -> (x-y=w1127:i32)
        n162 = Number To Decimal String(number=w1119) -> (decimal integer string=w1118:string)  [unwired: 1 in]
        n163 = Number To Decimal String(number=w1123) -> (decimal integer string=w1122:string)  [unwired: 1 in]
        n164 = Number To Decimal String(number=w1127) -> (decimal integer string=w1126:string)  [unwired: 1 in]
        n165 = Build Array(w1117, w1113, w1116, w1115, w1114, w1111, w1131, w1130, w1118, w1120, w1121, w1122, w1124, w1125, w1126, w1128) -> (w1098:string[])
        "appended array 4" <- w1098
        n166 = Insert Into Array(array=w1134, new element=w1098) -> (w1135:string[][])  [unwired: 2 in]
      }
      n167 = call-poly <vilib>:"DB Tools Free Object.vi"("error in (no error)"=w1082, "recordset reference"=w1086) -> ("error out"=w1081:errorcluster, "connection reference"=w1085:T1)  [unwired: 8 in]
      n168 = call <vilib>:"DB Tools Close Connection.vi"("error in (no error)"=w1081, "connection reference"=w1085) -> ("error out"=→"error out 5":errorcluster)  [unwired: 5 in]
      n169 = Array Size(array=w1058) -> ()  [unwired: 1 out]
      n170 = Add Array Elements(numeric array=w1039) -> (sum=w1033:i32)
      n171 = Add Array Elements(numeric array=w1040) -> (sum=w1034:i32)
      n172 = Add Array Elements(numeric array=w1030) -> (sum=w1026:i32)
      n173 = Add Array Elements(numeric array=w1021) -> (sum=w1019:i32)
      n174 = Add Array Elements(numeric array=w1029) -> (sum=w1025:i32)
      n175 = Add Array Elements(numeric array=w1022) -> (sum=w1020:i32)
      n176 = Add Array Elements(numeric array=w1051) -> (sum=w1046:i32)
      n177 = Add Array Elements(numeric array=w1050) -> (sum=w1045:i32)
      n178 = Subtract(x=w1020, y=w1019) -> (x-y=w1018:i32)
      n179 = Subtract(x=w1026, y=w1025) -> (x-y=w1023:i32)
      n180 = Subtract(x=w1046, y=w1045) -> (x-y=w1038:i32)
      n181 = Subtract(x=w1034, y=w1033) -> (x-y=w1031:i32)
      n182 = Number To Decimal String(number=w1033) -> (decimal integer string=w1035:string)  [unwired: 1 in]
      n183 = Number To Decimal String(number=w1031) -> (decimal integer string=w1032:string)  [unwired: 1 in]
      n184 = Number To Decimal String(number=w1026) -> (decimal integer string=w1028:string)  [unwired: 1 in]
      n185 = Number To Decimal String(number=w1025) -> (decimal integer string=w1027:string)  [unwired: 1 in]
      n186 = Number To Decimal String(number=w1023) -> (decimal integer string=w1024:string)  [unwired: 1 in]
      n187 = Number To Decimal String(number=w1018) -> (decimal integer string=w1015:string)  [unwired: 1 in]
      n188 = Number To Decimal String(number=w1046) -> (decimal integer string=w1048:string)  [unwired: 1 in]
      n189 = Number To Decimal String(number=w1045) -> (decimal integer string=w1047:string)  [unwired: 1 in]
      n190 = Number To Decimal String(number=w1034) -> (decimal integer string=w1037:string)  [unwired: 1 in]
      n191 = Number To Decimal String(number=w1020) -> (decimal integer string=w1017:string)  [unwired: 1 in]
      n192 = Number To Decimal String(number=w1019) -> (decimal integer string=w1016:string)  [unwired: 1 in]
      n193 = Number To Decimal String(number=w1038) -> (decimal integer string=w1044:string)  [unwired: 1 in]
      n194 = Build Array(w1049, w1049, "Total :" ("element"), w1048, w1047, w1044, w1037, w1035, w1032, w1028, w1027, w1024, w1017, w1016, w1015, "") -> (w1043:string[])
      n195 = Insert Into Array(array=w1042, new element=w1043) -> (w1041:string[][])  [unwired: 2 in]
      n196 = local write "Table Control 3"(w1041) -> ()
    }
    frame #3 {
      w1555 = ""
      n197 = call-poly <vilib>:"DB Tools Open Connection.vi"("connection information"=path "c:/m100/data/m100.dsn") -> ("error out"=w1590:errorcluster, "connection reference"=w1594:T1)  [unwired: 7 in]
      n198 = call-poly <vilib>:"DB Tools Execute Query.vi"("error in (no error)"=w1590, "SQL query"="select distinct d.mt_customer,d.mt_package,d.mt_device,\n      (select isnull(sum(a.mt_pass),0) from m100.dbo.mt_data a\n      where a.mt_customer=d.mt_customer\n        and a.mt_package=d.mt_package\n        and a.mt_device=d.mt_device\n        and a.mt_machine like 'QAMT%'\n        and a.mt_rc_no like 'A%' \n        and CONVERT(varchar,a.mt_end,111)=convert(varchar,getdate()-4,111)\n        and a.mt_shift='©]') as shifta,\n        (select isnull(sum(a.mt_total),0) from m100.dbo.mt_data a\n      where a.mt_customer=d.mt_customer\n        and a.mt_package=d.mt_package\n        and a.mt_device=d.mt_device\n        and a.mt_machine like 'QAMT%'\n        and a.mt_rc_no like 'A%' \n        and CONVERT(varchar,a.mt_end,111)=convert(varchar,getdate()-4,111)\n        and a.mt_shift='©]') as shifta1,\n        (select isnull(sum(b.mt_pass),0) from m100.dbo.mt_data b\n      where b.mt_customer=d.mt_customer\n        and b.mt_package=d.mt_package\n       and b.mt_device=d.mt_device\n        and b.mt_machine like 'QAMT%'\n        and b.mt_rc_no like 'A%' \n        and CONVERT(varchar,b.mt_end,111)=convert(varchar,getdate()-4,111)\n        and b.mt_shift='¦­') as shiftb,\n        (select isnull(sum(b.mt_total),0) from m100.dbo.mt_data b\n      where b.mt_customer=d.mt_customer\n        and b.mt_package=d.mt_package\n        and b.mt_device=d.mt_device\n        and b.mt_machine like 'QAMT%'\n        and b.mt_rc_no like 'A%' \n        and CONVERT(varchar,b.mt_end,111)=convert(varchar,getdate()-4,111)\n        and b.mt_shift='¦­') as shiftb1,\n        (select isnull(sum(c.mt_pass),0) from m100.dbo.mt_data c\n      where c.mt_customer=d.mt_customer\n        and c.mt_package=d.mt_package\n        and c.mt_device=d.mt_device\n        and c.mt_machine like 'QAMT%'\n        and c.mt_rc_no like 'A%' \n        and CONVERT(varchar,c.mt_end,111)=convert(varchar,getdate()-4,111)\n        and c.mt_shift='¤¤') as shiftc,\n        (select isnull(sum(c.mt_total),0) from m100.dbo.mt_data c\n      where c.mt_customer=d.mt_customer\n        and c.mt_package=d.mt_package\n        and c.mt_device=d.mt_device\n        and c.mt_machine like 'QAMT%'\n        and c.mt_rc_no like 'A%' \n        and CONVERT(varchar,c.mt_end,111)=convert(varchar,getdate()-4,111)\n        and c.mt_shift='¤¤') as shiftc1,\n        SUM(mt_pass),SUM(mt_total),master.dbo.GetEntityNameFromDateToDate(d.mt_customer,d.mt_package,d.mt_device,CONVERT(varchar,GETDATE()-4,111),CONVERT(varchar,GETDATE()-4,111))\n  FROM [m100].[dbo].[mt_data] d\n  WHERE d.mt_customer='MST'\n    and d.mt_machine like 'QAMT%'\n    AND CONVERT(varchar,d.mt_end,111)=convert(varchar,getdate()-4,111)\n    and d.mt_pass > 0 and d.mt_rc_no like 'A%'\n      group by d.mt_customer,d.mt_package,d.mt_device", "connection reference"=w1594) -> ("error out"=w1589:errorcluster, "recordset reference"=w1593:T2)  [unwired: 5 in]
      n199 = call-poly <vilib>:"DB Tools Fetch Recordset Data.vi"("error in (no error)"=w1589, "recordset reference"=w1593) -> ("error out"=w1588:errorcluster, "recordset data"=w1558:variant[][], "recordset reference out"=w1592:T2)  [unwired: 3 in]
      "recordset data 5" <- w1558
      n200 = Index Array(array=w1558, index (col) #1=0 ("index (row)"), index (col) #2=1 ("index (col)"), index (col) #3=2 ("disabled index (col)"), index (col) #4=3 ("index (col)"), index (col) #5=4 ("index (col)"), index (col) #6=5 ("index (col)"), index (col) #7=6 ("index (col)"), index (col) #8=7 ("index (col)"), index (col) #9=8 ("index (col)"), index (col) #10=9 ("index (col)"), index (col) #11=10 ("index (col)"), index (col) #12=11 ("index (col)")) -> (element #1=w1562:variant[], element #2=w1561:variant[], element #3=w1575:variant[], element #4=w1574:variant[], element #5=w1573:variant[], element #6=w1572:variant[], element #7=w1571:variant[], element #8=w1570:variant[], element #9=w1569:variant[], element #10=w1568:variant[], element #11=w1567:variant[], element #12=w1566:variant[])  [unwired: 12 in]
      n201 = for {
        tunnel: w1575 -> [w1614] mode=indexing
        tunnel: w1574 -> [w1613] mode=indexing
        tunnel: w1573 -> [w1612] mode=indexing
        tunnel: w1572 -> [w1611] mode=indexing
        tunnel: w1571 -> [w1610] mode=indexing
        tunnel: w1570 -> [w1609] mode=indexing
        tunnel: w1569 -> [w1608] mode=indexing
        tunnel: w1568 -> [w1607] mode=indexing
        tunnel: w1567 -> [w1606] mode=indexing
        tunnel: w1566 -> [w1605] mode=indexing
        tunnel: [w1641] -> w1548
        shift-right: [w1641] -> w1564
        shift-left: string[][] [] ("array") -> [w1640]
        tunnel: w1562 -> [w1616] mode=indexing
        tunnel: w1561 -> [w1615] mode=indexing
        tunnel: [w1603] -> w1557 mode=indexing
        tunnel: [w1602] -> w1556 mode=indexing
        tunnel: [w1601] -> w1546 mode=indexing
        tunnel: [w1600] -> w1545 mode=indexing
        tunnel: [w1599] -> w1536 mode=indexing
        tunnel: [w1598] -> w1535 mode=indexing
        tunnel: [w1597] -> w1528 mode=indexing
        tunnel: [w1596] -> w1527 mode=indexing
        w1639 = ""
        n202 = xnode "Database Variant To Data"("database variant"=w1613, "type"=0) -> ("data"=w1603:i32)  [unwired: 1 in, 1 out]
        n203 = xnode "Database Variant To Data"("database variant"=w1610, "type"=w1603) -> ("data"=w1600:i32)  [unwired: 1 in, 1 out]
        n204 = xnode "Database Variant To Data"("database variant"=w1607, "type"=w1600) -> ("data"=w1597:i32)  [unwired: 1 in, 1 out]
        n205 = xnode "Database Variant To Data"("database variant"=w1614, "type"=w1639) -> ("data"=w1622:string)  [unwired: 1 in, 1 out]
        n206 = xnode "Database Variant To Data"("database variant"=w1611, "type"=w1603) -> ("data"=w1601:i32)  [unwired: 1 in, 1 out]
        n207 = xnode "Database Variant To Data"("database variant"=w1608, "type"=w1600) -> ("data"=w1598:i32)  [unwired: 1 in, 1 out]
        n208 = xnode "Database Variant To Data"("database variant"=w1605, "type"="") -> ("data"=w1634:string)  [unwired: 1 in, 1 out]
        n209 = xnode "Database Variant To Data"("database variant"=w1609, "type"=w1600) -> ("data"=w1599:i32)  [unwired: 1 in, 1 out]
        n210 = xnode "Database Variant To Data"("database variant"=w1615, "type"=w1639) -> ("data"=w1619:string)  [unwired: 1 in, 1 out]
        n211 = Number To Decimal String(number=w1603) -> (decimal integer string=w1621:string)  [unwired: 1 in]
        n212 = xnode "Database Variant To Data"("database variant"=w1612, "type"=w1603) -> ("data"=w1602:i32)  [unwired: 1 in, 1 out]
        n213 = xnode "Database Variant To Data"("database variant"=w1606, "type"=w1597) -> ("data"=w1596:i32)  [unwired: 1 in, 1 out]
        n214 = xnode "Database Variant To Data"("database variant"=w1616, "type"=w1639) -> ("data"=w1623:string)  [unwired: 1 in, 1 out]
        n215 = Number To Decimal String(number=w1602) -> (decimal integer string=w1620:string)  [unwired: 1 in]
        n216 = Number To Decimal String(number=w1601) -> (decimal integer string=w1637:string)  [unwired: 1 in]
        n217 = Number To Decimal String(number=w1600) -> (decimal integer string=w1636:string)  [unwired: 1 in]
        n218 = Number To Decimal String(number=w1597) -> (decimal integer string=w1630:string)  [unwired: 1 in]
        n219 = Number To Decimal String(number=w1599) -> (decimal integer string=w1626:string)  [unwired: 1 in]
        n220 = Number To Decimal String(number=w1598) -> (decimal integer string=w1627:string)  [unwired: 1 in]
        n221 = Number To Decimal String(number=w1596) -> (decimal integer string=w1631:string)  [unwired: 1 in]
        n222 = Subtract(x=w1603, y=w1602) -> (x-y=w1618:i32)
        n223 = Number To Decimal String(number=w1618) -> (decimal integer string=w1617:string)  [unwired: 1 in]
        n224 = Subtract(x=w1601, y=w1600) -> (x-y=w1625:i32)
        n225 = Subtract(x=w1599, y=w1598) -> (x-y=w1629:i32)
        n226 = Subtract(x=w1597, y=w1596) -> (x-y=w1633:i32)
        n227 = Number To Decimal String(number=w1625) -> (decimal integer string=w1624:string)  [unwired: 1 in]
        n228 = Number To Decimal String(number=w1629) -> (decimal integer string=w1628:string)  [unwired: 1 in]
        n229 = Number To Decimal String(number=w1633) -> (decimal integer string=w1632:string)  [unwired: 1 in]
        n230 = Build Array(w1623, w1619, w1622, w1621, w1620, w1617, w1637, w1636, w1624, w1626, w1627, w1628, w1630, w1631, w1632, w1634) -> (w1604:string[])
        "appended array 5" <- w1604
        n231 = Insert Into Array(array=w1640, new element=w1604) -> (w1641:string[][])  [unwired: 2 in]
      }
      n232 = call-poly <vilib>:"DB Tools Free Object.vi"("error in (no error)"=w1588, "recordset reference"=w1592) -> ("error out"=w1587:errorcluster, "connection reference"=w1591:T1)  [unwired: 8 in]
      n233 = call <vilib>:"DB Tools Close Connection.vi"("error in (no error)"=w1587, "connection reference"=w1591) -> ("error out"=→"error out 6":errorcluster)  [unwired: 5 in]
      n234 = Array Size(array=w1564) -> ()  [unwired: 1 out]
      n235 = Add Array Elements(numeric array=w1545) -> (sum=w1539:i32)
      n236 = Add Array Elements(numeric array=w1546) -> (sum=w1540:i32)
      n237 = Add Array Elements(numeric array=w1536) -> (sum=w1532:i32)
      n238 = Add Array Elements(numeric array=w1527) -> (sum=w1525:i32)
      n239 = Add Array Elements(numeric array=w1535) -> (sum=w1531:i32)
      n240 = Add Array Elements(numeric array=w1528) -> (sum=w1526:i32)
      n241 = Add Array Elements(numeric array=w1557) -> (sum=w1552:i32)
      n242 = Add Array Elements(numeric array=w1556) -> (sum=w1551:i32)
      n243 = Subtract(x=w1526, y=w1525) -> (x-y=w1524:i32)
      n244 = Subtract(x=w1532, y=w1531) -> (x-y=w1529:i32)
      n245 = Subtract(x=w1552, y=w1551) -> (x-y=w1544:i32)
      n246 = Subtract(x=w1540, y=w1539) -> (x-y=w1537:i32)
      n247 = Number To Decimal String(number=w1539) -> (decimal integer string=w1541:string)  [unwired: 1 in]
      n248 = Number To Decimal String(number=w1537) -> (decimal integer string=w1538:string)  [unwired: 1 in]
      n249 = Number To Decimal String(number=w1532) -> (decimal integer string=w1534:string)  [unwired: 1 in]
      n250 = Number To Decimal String(number=w1531) -> (decimal integer string=w1533:string)  [unwired: 1 in]
      n251 = Number To Decimal String(number=w1529) -> (decimal integer string=w1530:string)  [unwired: 1 in]
      n252 = Number To Decimal String(number=w1524) -> (decimal integer string=w1521:string)  [unwired: 1 in]
      n253 = Number To Decimal String(number=w1552) -> (decimal integer string=w1554:string)  [unwired: 1 in]
      n254 = Number To Decimal String(number=w1551) -> (decimal integer string=w1553:string)  [unwired: 1 in]
      n255 = Number To Decimal String(number=w1540) -> (decimal integer string=w1543:string)  [unwired: 1 in]
      n256 = Number To Decimal String(number=w1526) -> (decimal integer string=w1523:string)  [unwired: 1 in]
      n257 = Number To Decimal String(number=w1525) -> (decimal integer string=w1522:string)  [unwired: 1 in]
      n258 = Number To Decimal String(number=w1544) -> (decimal integer string=w1550:string)  [unwired: 1 in]
      n259 = Build Array(w1555, w1555, "Total :" ("element"), w1554, w1553, w1550, w1543, w1541, w1538, w1534, w1533, w1530, w1523, w1522, w1521, "") -> (w1549:string[])
      n260 = Insert Into Array(array=w1548, new element=w1549) -> (w1547:string[][])  [unwired: 2 in]
      n261 = local write "Table Control 4"(w1547) -> ()
    }
    frame #4 {
      w2046 = "macro1" ("macro name")
      w2120 = "MSTDailyReport"
      w2062 = string[] ["Customer", "Package", "Device", "Total", "Pass", "Fail", "Total", "Pass", "Fail", "Total", "Pass", "Fail", "Total", "Pass", "Fail", "Machine"] ("row headers")
      w2042 = cluster{"row":i32, "column":i32} {"row"=0, "column"=0} ("end (-1, -1)")
      w2137 = T3."Excel"  # Report Type
      # "Simulate UUT Testing"
      n262 = call <vilib>:"New Report.vi"("report type"=w2137, "template (empty)"="Report Template") -> ("report out"=w2133:refnum<class "NI_report.lvclass">, "error out"=w2132:errorcluster)  [unwired: 12 in]
      n263 = call <vilib>:"Excel Get Worksheet.vi"("report in"=w2133, "worksheet index (0)"=0, "error in (no error)"=w2132) -> ("report out"=w2037:refnum<class "NI_report.lvclass">, "error out"=w2036:errorcluster)  [unwired: 11 in]
      n264 = Get Date/Time In Seconds() -> (seconds since 1Jan1904=w2126:timestamp)
      n265 = Subtract(x=w2126, y=86400) -> (x-y=w2033:timestamp)
      n266 = Format Date/Time String(time format string (%c)="%Y-%m-%d", seconds (now)=w2033) -> (date/time string=w2031:string)  [unwired: 1 in]
      n267 = call <vilib>:"Excel Rename Worksheet.vi"("report in"=w2037, "worksheet name (\"\")"=w2031, "error in (no error)"=w2036) -> ("report out"=w2035:refnum<class "NI_report.lvclass">, "error out"=w2034:errorcluster)  [unwired: 11 in]
      n268 = call-poly <vilib>:"Append Table to Report.vi"("report in"=w2035, "column headers"=w2062, "text data"="Table Control", "error in (no error)"=w2034) -> ("report out"=w2135:refnum<class "NI_report.lvclass">, "error out"=w2134:errorcluster)  [unwired: 8 in, 2 out]
      n269 = Get Date/Time String(seconds (now)=w2033) -> (date string=w2118:string)  [unwired: 2 in, 1 out]
      n270 = call <vilib>:"Excel Insert Cells.vi"("report in"=w2135, "error in (no error)"=w2134) -> ("report out"=w2131:refnum<class "NI_report.lvclass">, "error out"=w2130:errorcluster)  [unwired: 12 in]
      n271 = Concatenate Strings("Date :" ("string"), w2118, "  00:00 - 24:00" ("string")) -> (w2128:string)
      n272 = call <vilib>:"Excel Easy Text.vi"("report in"=w2131, "text"=w2128, "start (-1, -1)"=w2042, "error in (no error)"=w2130) -> ("report out"=w2115:refnum<class "NI_report.lvclass">, "error out"=w2114:errorcluster)  [unwired: 7 in, 3 out]
      n273 = call <vilib>:"Excel Run Macro.vi"("report in"=w2115, "macro name"=w2046, "error in (no error)"=w2114) -> ("report out"=w2113:refnum<class "NI_report.lvclass">, "error out"=w2112:errorcluster)  [unwired: 10 in, 1 out]
      n274 = Get Date/Time In Seconds() -> (seconds since 1Jan1904=w2104:timestamp)
      n275 = call <vilib>:"Excel Get Worksheet.vi"("report in"=w2113, "worksheet index (0)"=1, "error in (no error)"=w2112) -> ("report out"=w2110:refnum<class "NI_report.lvclass">, "error out"=w2109:errorcluster)  [unwired: 11 in]
      n276 = Subtract(x=w2104, y=172800) -> (x-y=w2094:timestamp)
      n277 = Get Date/Time String(seconds (now)=w2094) -> (date string=w2095:string)  [unwired: 2 in, 1 out]
      n278 = call-poly <vilib>:"Append Table to Report.vi"("report in"=w2110, "column headers"=w2062, "text data"="Table Control 2", "error in (no error)"=w2109) -> ("report out"=w2107:refnum<class "NI_report.lvclass">, "error out"=w2106:errorcluster)  [unwired: 8 in, 2 out]
      n279 = call <vilib>:"Excel Insert Cells.vi"("report in"=w2107, "error in (no error)"=w2106) -> ("report out"=w2101:refnum<class "NI_report.lvclass">, "error out"=w2100:errorcluster)  [unwired: 12 in]
      n280 = Format Date/Time String(time format string (%c)="%Y-%m-%d", seconds (now)=w2094) -> (date/time string=w2092:string)  [unwired: 1 in]
      n281 = Concatenate Strings("Date :" ("string"), w2095, "  00:00 - 24:00" ("string")) -> (w2091:string)
      n282 = call <vilib>:"Excel Easy Text.vi"("report in"=w2101, "text"=w2091, "start (-1, -1)"=w2042, "error in (no error)"=w2100) -> ("report out"=w2099:refnum<class "NI_report.lvclass">, "error out"=w2098:errorcluster)  [unwired: 7 in, 3 out]
      n283 = call <vilib>:"Excel Run Macro.vi"("report in"=w2099, "macro name"=w2046, "error in (no error)"=w2098) -> ("report out"=w2097:refnum<class "NI_report.lvclass">, "error out"=w2096:errorcluster)  [unwired: 10 in, 1 out]
      n284 = call <vilib>:"Excel Rename Worksheet.vi"("report in"=w2097, "worksheet name (\"\")"=w2092, "error in (no error)"=w2096) -> ("report out"=w2069:refnum<class "NI_report.lvclass">, "error out"=w2068:errorcluster)  [unwired: 11 in]
      n285 = call <vilib>:"Excel Get Worksheet.vi"("report in"=w2069, "worksheet index (0)"=2, "error in (no error)"=w2068) -> ("report out"=w2089:refnum<class "NI_report.lvclass">, "error out"=w2088:errorcluster)  [unwired: 11 in]
      n286 = Get Date/Time In Seconds() -> (seconds since 1Jan1904=w2083:timestamp)
      n287 = call-poly <vilib>:"Append Table to Report.vi"("report in"=w2089, "column headers"=w2062, "text data"="Table Control 3", "error in (no error)"=w2088) -> ("report out"=w2086:refnum<class "NI_report.lvclass">, "error out"=w2085:errorcluster)  [unwired: 8 in, 2 out]
      n288 = Subtract(x=w2083, y=259200) -> (x-y=w2073:timestamp)
      n289 = Get Date/Time String(seconds (now)=w2073) -> (date string=w2074:string)  [unwired: 2 in, 1 out]
      n290 = call <vilib>:"Excel Insert Cells.vi"("report in"=w2086, "error in (no error)"=w2085) -> ("report out"=w2080:refnum<class "NI_report.lvclass">, "error out"=w2079:errorcluster)  [unwired: 12 in]
      n291 = Concatenate Strings("Date :" ("string"), w2074, "  00:00 - 24:00" ("string")) -> (w2070:string)
      n292 = call <vilib>:"Excel Easy Text.vi"("report in"=w2080, "text"=w2070, "start (-1, -1)"=w2042, "error in (no error)"=w2079) -> ("report out"=w2078:refnum<class "NI_report.lvclass">, "error out"=w2077:errorcluster)  [unwired: 7 in, 3 out]
      n293 = Format Date/Time String(time format string (%c)="%Y-%m-%d", seconds (now)=w2073) -> (date/time string=w2071:string)  [unwired: 1 in]
      n294 = call <vilib>:"Excel Run Macro.vi"("report in"=w2078, "macro name"=w2046, "error in (no error)"=w2077) -> ("report out"=w2076:refnum<class "NI_report.lvclass">, "error out"=w2075:errorcluster)  [unwired: 10 in, 1 out]
      n295 = call <vilib>:"Excel Rename Worksheet.vi"("report in"=w2076, "worksheet name (\"\")"=w2071, "error in (no error)"=w2075) -> ("report out"=w2067:refnum<class "NI_report.lvclass">, "error out"=w2066:errorcluster)  [unwired: 11 in]
      n296 = Get Date/Time In Seconds() -> (seconds since 1Jan1904=w2055:timestamp)
      n297 = call <vilib>:"Excel Get Worksheet.vi"("report in"=w2067, "worksheet index (0)"=3, "error in (no error)"=w2066) -> ("report out"=w2064:refnum<class "NI_report.lvclass">, "error out"=w2063:errorcluster)  [unwired: 11 in]
      n298 = Subtract(x=w2055, y=345600) -> (x-y=w2052:timestamp)
      n299 = Get Date/Time String(seconds (now)=w2052) -> (date string=w2050:string)  [unwired: 2 in, 1 out]
      n300 = Concatenate Strings("Date :" ("string"), w2050, "  00:00 - 24:00" ("string")) -> (w2049:string)
      n301 = call-poly <vilib>:"Append Table to Report.vi"("report in"=w2064, "column headers"=w2062, "text data"="Table Control 4", "error in (no error)"=w2063) -> ("report out"=w2060:refnum<class "NI_report.lvclass">, "error out"=w2059:errorcluster)  [unwired: 8 in, 2 out]
      n302 = call <vilib>:"Excel Insert Cells.vi"("report in"=w2060, "error in (no error)"=w2059) -> ("report out"=w2058:refnum<class "NI_report.lvclass">, "error out"=w2057:errorcluster)  [unwired: 12 in]
      n303 = Format Date/Time String(time format string (%c)="%Y-%m-%d", seconds (now)=w2052) -> (date/time string=w2043:string)  [unwired: 1 in]
      n304 = call <vilib>:"Excel Easy Text.vi"("report in"=w2058, "text"=w2049, "start (-1, -1)"=w2042, "error in (no error)"=w2057) -> ("report out"=w2048:refnum<class "NI_report.lvclass">, "error out"=w2047:errorcluster)  [unwired: 7 in, 3 out]
      n305 = call <vilib>:"Excel Run Macro.vi"("report in"=w2048, "macro name"=w2046, "error in (no error)"=w2047) -> ("report out"=w2045:refnum<class "NI_report.lvclass">, "error out"=w2044:errorcluster)  [unwired: 10 in, 1 out]
      n306 = call "DateTimeToStringDateWith0.vi"("time stamp"=w2033) -> ("Dateyyyymmdd"=w2121:string)  [unwired: 9 in, 1 out]
      n307 = call <vilib>:"Excel Rename Worksheet.vi"("report in"=w2045, "worksheet name (\"\")"=w2043, "error in (no error)"=w2044) -> ("report out"=w2030:refnum<class "NI_report.lvclass">, "error out"=w2028:errorcluster)  [unwired: 11 in]
      n308 = Concatenate Strings(w2120, w2121, ".xls" ("string")) -> (w2122:string)
      n309 = Concatenate Strings(w2120, w2121) -> ()  [unwired: 1 out]
      n310 = call <vilib>:"Excel Get Worksheet.vi"("report in"=w2030, "worksheet index (0)"=0, "error in (no error)"=w2028) -> ("report out"=w2029:refnum<class "NI_report.lvclass">, "error out"=w2027:errorcluster)  [unwired: 11 in]
      n311 = Build Path(base path=path "o:/monitor/report", name or relative path=w2122) -> (appended path=w2119:path)
      n312 = call-dynamic "Save Report to File.vi"("report in"=w2029, "report file path"=w2119, "error in (no error)"=w2027) -> ("report out"=w2039:refnum<class "NI_report.lvclass">, "error out"=w2038:errorcluster)  [unwired: 11 in]
      n313 = call-dynamic "Dispose Report.vi"("report in"=w2039, "save changes? (F)"=FALSE, "error in (no error)"=w2038) -> ("error out"=→"error out 4":errorcluster)  [unwired: 12 in]
    }
    frame #5 {
      n314 = Index Array(array=w2141) -> (element=w2140:i32)  [unwired: 1 in]
      n315 = Greater?(x=w2140, y=1) -> (0:w2138:bool)
      n316 = case shown="True" w2138 {
        tunnel: w2143 -> [_ w2146]
        tunnel: w2142 -> [_ w2145]
        frame False {
        }
        frame True {
          (unwired) string[] ["yyliao@ptse.com.tw", "p110@ptse.com.tw", "s100@ptse.com.tw", "m110@ptse.com.tw", "e100@ptse.com.tw", "eric_fan@ptse.com.tw", "saulwang@ptse.com.tw", "jtwu@ptse.com.tw", "Allonsite@mstarsemi.com", "hank.huang@mstarsemi.com", "jerry.fu@mstarsemi.com", "Allpeusers@mstarsemi.com", "stanley.wang@mstarsemi.com", "sam-cs.lin@mstarsemi.com", "AllPCUsers@mstarsemi.com", "joey.hsien@mstarsemi.com"] ("recipients")
          (unwired) "***** MST Daily Report from PTS *****" ("subject ([No Subject])")
          (unwired) string[] ["yyliao@ptse.com.tw"] ("recipients")
          n317 = Current VI's Path() -> (path=w2150:path)
          n318 = Strip Path(path=w2150) -> (name=w2149:string)  [unwired: 1 out]
          n319 = Match Pattern(string=w2149, regular expression=".vi") -> (before substring=w2147:string)  [unwired: 1 in, 3 out]
          n320 = call "MailMessage.vi"("AddSubject"=w2145, "message"="Dear sirs,\n\nAttached the Daily Report for your information,\n\nBest Regards,\n\n", "file path"=w2146, "program"=w2147) -> ()  [unwired: 8 in]
        }
      }
    }
    frame #6 {
      n321 = Quit LabVIEW() -> ()  [unwired: 1 in]
    }
  }
